vi "a前面板.vi"() -> ()   [LabVIEW 2018]
uses:
  D:/Program Files (x86)/National Instruments/LabVIEW 2018/examples/Instrument IO/Serial/support/Serial - Settings.ctl
  <vilib>/Instr/_visa.llb/VISA Configure Serial Port (Instr).vi
panel:
  out "s4":dbl format="%#.2f"
  out "s3":dbl format="%#.2f"
  out "s2":dbl format="%#.2f"
  out "s1":dbl format="%#.2f"
  out "X体横向位移2 2":dbl
  out "X体横向位移1 2":dbl
  in  "调零":bool
  out "调零后累计流量":dbl format="%.2f"
  out "瞬时流量 2":dbl format="%.2f"
  out "周向转动摩擦力2":dbl format="%#.3f"
  out "周向转动摩擦力1":dbl format="%#.3f"
  out "横向拉压力2":dbl
  out "横向拉压力1":dbl
  out "累计流量 2":dbl
  in  "VISA资源名称":refnum<visa-resource-name>="COM7"
  in  "读取前延时(ms)":u32=15
  out "响应":string
  out "读取的字节":u32
  in  "串口设置":T1={"波特率"=115200, "数据位"=8, "校验"=enum."None", "停止位"=10, "流控制"=0} {"流控制" items=["无"=0, "XON/XOFF"=1, "RTS/CTS"=2, "DTR/DSR"=4]; "停止位" items=["1.0"=10, "1.5"=15, "2.0"=20]; "数据位" min=5 max=8 step=1; "波特率" items=["75"=75, "110"=110, "134"=134, "150"=150, "300"=300, "600"=600, "1200"=1200, "1800"=1800, "2400"=2400, "4800"=4800, "7200"=7200, "9600"=9600, "14400"=14400, "19200"=19200, "28800"=28800, "38400"=38400, "56000"=56000, "57600"=57600, "115200"=115200, "128000"=128000, "230400"=230400]}
  out "连接的字符串 3":string
  out "连接的字符串 4":string
  out "瞬时流量":dbl format="%#.6f"
  out "总累计流量":dbl
  out "字符串 3":string
  out "字符串 2":string
  out "布尔 2":bool
  out "减压后气压Mpa":dbl format="%#.2f"
  in  "显示选择":bool
  out "选项卡控件":enum32{"操作面板", "数据显示面板"}(tab)
  in  "球阀预调确认":bool
  in  "球阀开口预调":dbl=0.2 min=0.0 max=100.0
  out "球阀反馈值":dbl format="%#.1f"
  in  "试验结束":bool
  in  "手动模式":bool
  in  "cns":dbl min=0.0
  in  "放气":bool
  in  "放气延迟":bool
  in  "保压时间固定":bool
  in  "不保压":bool
  in  "程序停止":bool
  out "系统通讯正常":bool
  in  "p":dbl=0.1 min=0.1
  in  "I":dbl min=0.0 max=1.0
  in  "D":dbl min=0.0 max=1.0
  in  "紧急停止":bool
  in  "电磁阀1":bool
  in  "电磁阀2":bool
  in  "球阀开口度":dbl min=0.0 max=100.0
  in  "实验所需压力Mpa":dbl=0.2 min=0.0 max=0.9
  in  "时间s":dbl=1.0 min=1.0 max=21.0
  in  "全部放气":bool
  in  "容器放气":bool
  in  "数据保存 2":bool
  in  "结束保存 2":bool
  in  "采样频率 （HZ）":dbl=1.0 min=1.0 max=1000.0
  out "采样时间计时（s）":dbl
  in  "自动模式":bool
  in  "数据保存路径":path=path "D:/data/DATA"
  out "运行状态显示":string
  in  "刷新":bool
  out "气源气压Mpa":dbl format="%.2f"
  out "容器气压 Mpa":dbl format="%#.2f"
  out "容器压力2":dbl format="%#.2f"
  out "容器压力1":dbl format="%#.2f"
  out "电磁阀2":bool
  out "球阀":dbl format="%#.2f"
  out "电磁阀1":bool
  out "管道压力2":dbl format="%#.2f"
  out "管道压力1":dbl format="%#.2f"
  in  "调零":bool
  in  "紧急停止 2":bool
  out "运行状态显示 2":string
  in  "刷新 2":bool
  in  "选项卡控件 2":enum32{"管道压力1", "管道压力2", "容器压力1", "容器压力2"}(tab)
  out "管道气压1":dbl(graph)
  out "管道压力2":dbl(graph)
  out "容器压力1":dbl(graph)
  out "容器压力2":dbl(graph)
  in  "试验结束 2":bool
  out "周向转动摩擦力1t":dbl format="%#.2f"
  out "周向转动摩擦力2t":dbl format="%#.2f"
  out "横向拉压力1t":dbl format="%#_2f"
  out "横向拉压力2t":dbl format="%#_2f"
  in  "选项卡控件 5":enum32{"力", "位移"}(tab)
  in  "选项卡控件 3":T2(tab)
  out "横向拉压力1":dbl(graph)
  out "横向拉压力2":dbl(graph)
  out "周向转动摩擦力1":dbl(graph)
  out "周向转动摩擦力2":dbl(graph)
  in  "选项卡控件 4":enum32{"X体横向位移1", "X体横向位移2", "s1-s4"}(tab)
  out "X体横向位移1":dbl(graph)
  out "X体横向位移2":dbl(graph)
  out "位移s1-s4":dynamicdata(graph)
  out "X体横向位移1t":dbl format="%#.2f"
  out "X体横向位移2t":dbl format="%#.2f"
  out "s1t":dbl format="%#.2f"
  out "s2t":dbl format="%#.2f"
  out "s3t":dbl format="%#.2f"
  out "s4t":dbl format="%#.2f"
  # "弹筒适配空间模拟试验"
  # "数据保存"
  # "自动模式"
  # "手动模式"
  # "%"
  # "%"
  # "%"
  # "Mpa"
  # "Mpa"
  # "过滤器"
  # "过滤器"
  # "手动截止阀"
  # "储气罐"
  # "目标容器"
  # "干燥机"
  # "Mpa"
  # "手动截止阀"
  # "过滤器"
  # "减压阀"
  # "Mpa"
  # "单向阀"
  # "消音器"
  # "空压机"
  # "%"
  # "手动截止阀"
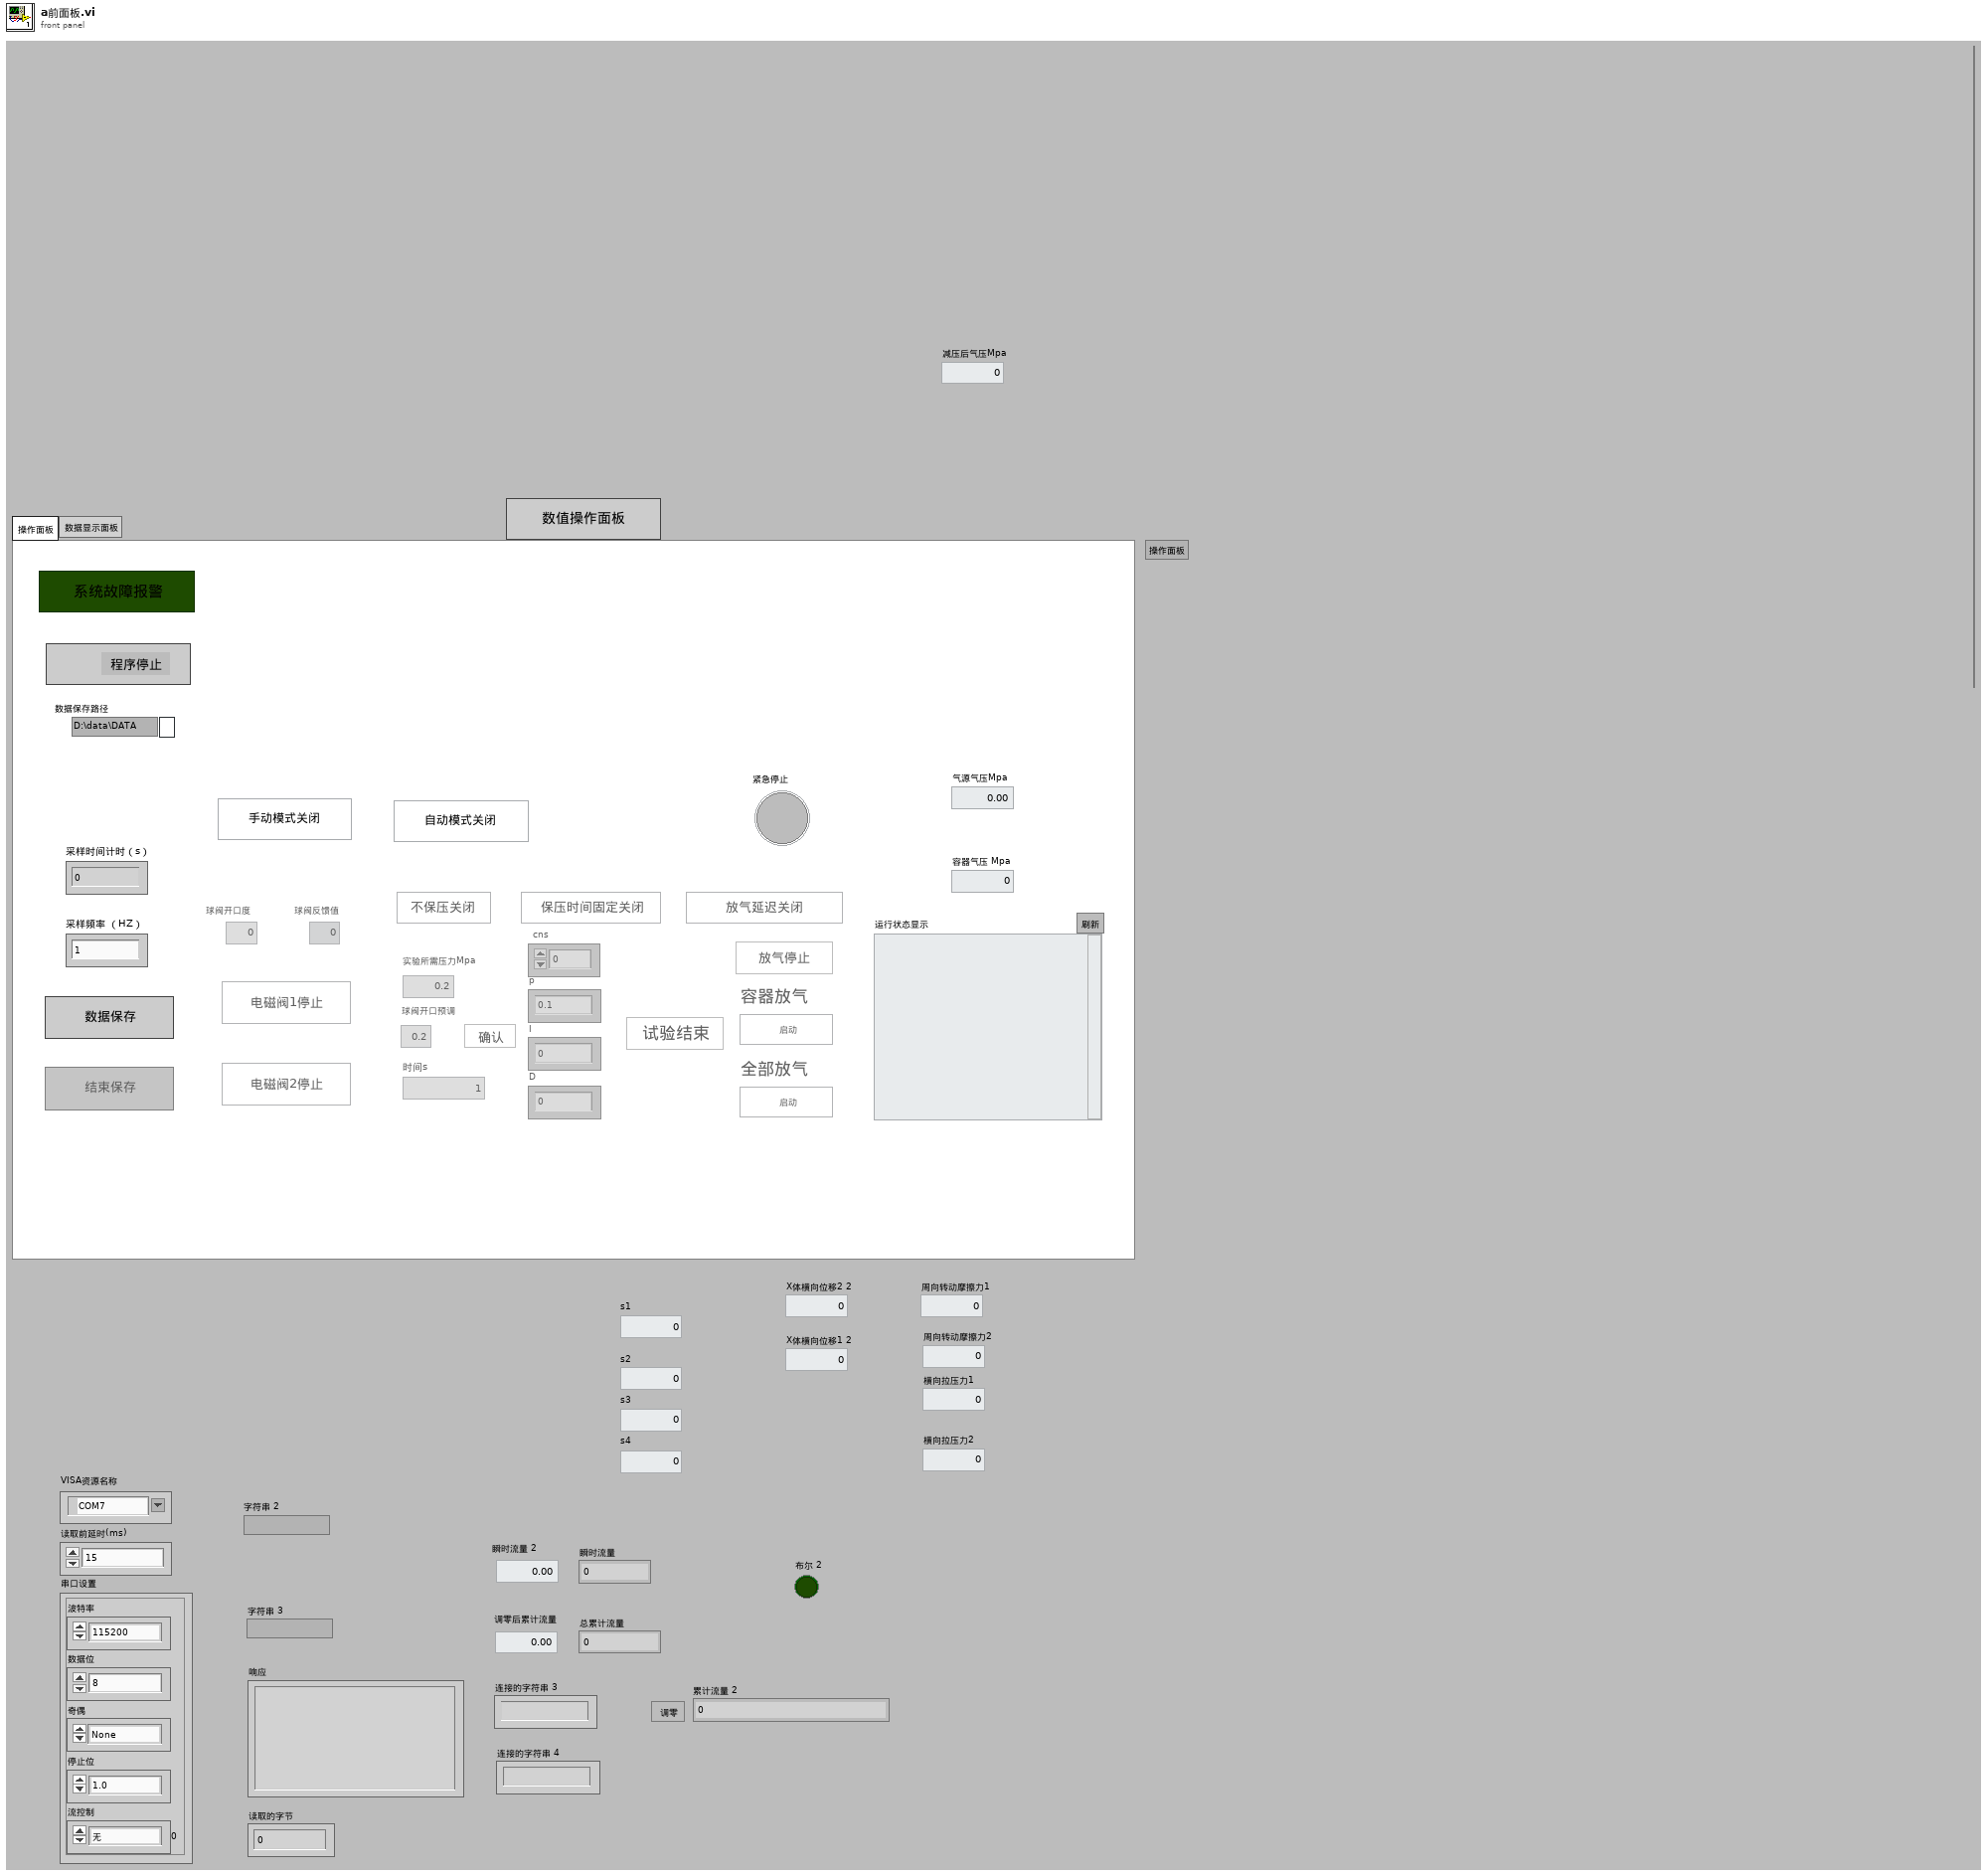
[diagram p1: front panel]
types:
  T1 = typedef "Serial - Settings.ctl" = cluster{"波特率":u32, "数据位":u16, "校验":enum16{"None", "Odd", "Even", "Mark", "Space"}, "停止位":u16, "流控制":u16}
  T2 = enum32{"横向拉压力1", "横向拉压力2", "周向转动摩擦力1", "周向转动摩擦力2"}
  T3 = enum16{"open", "replace", "create", "open or create", "replace or create", "replace or create with confirmation"}
  T4 = enum8{"Enabled", "Disabled", "Disabled and Grayed Out"}
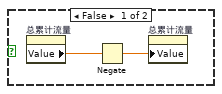
[diagram p3: hidden frame]
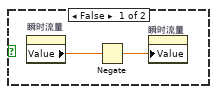
[diagram p4: hidden frame]
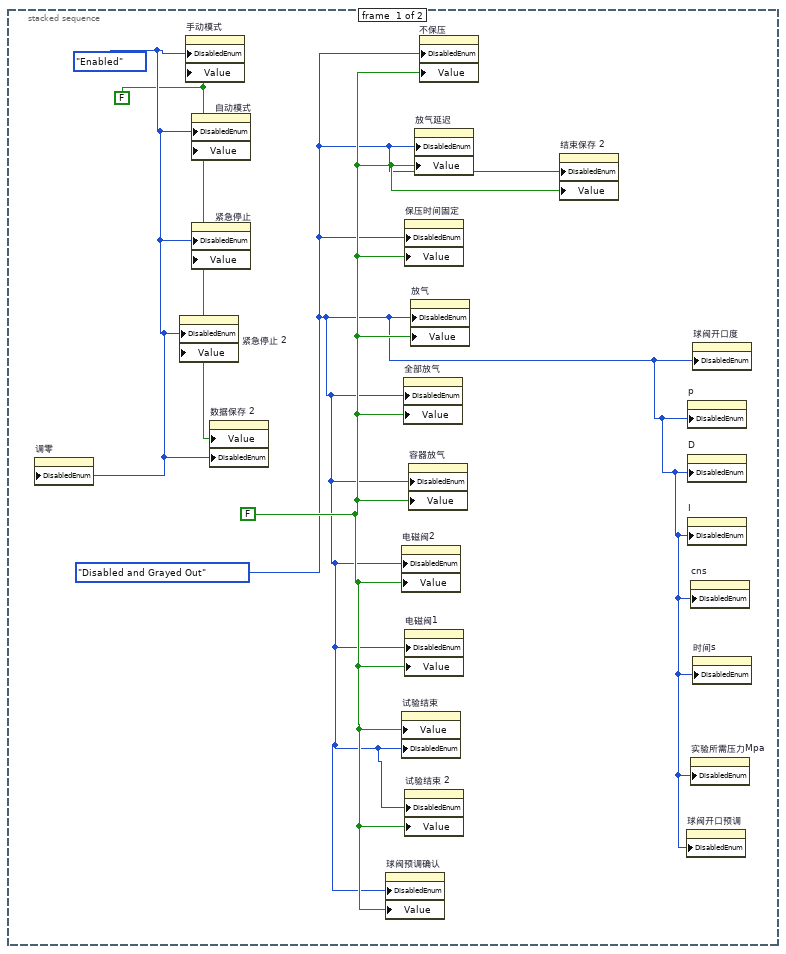
[diagram p5: hidden frame]
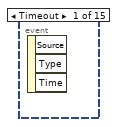
[diagram p6: hidden frame]
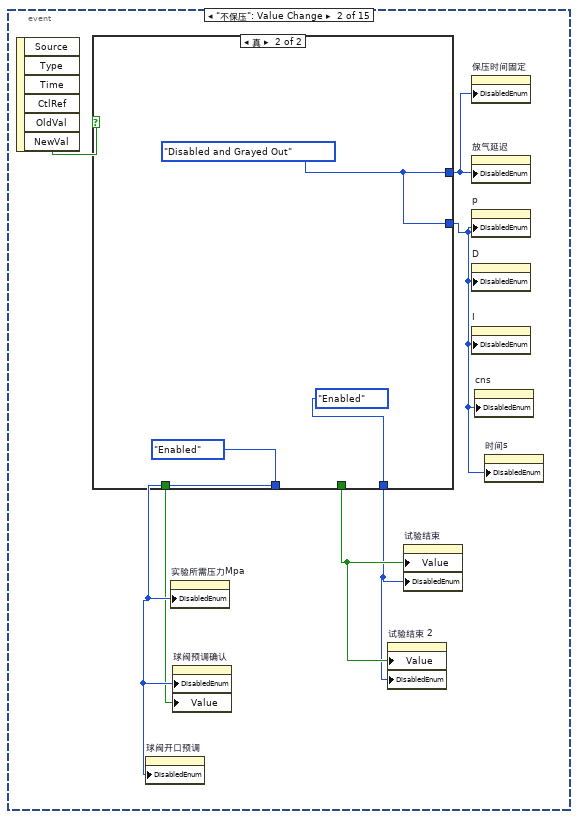
[diagram p7: hidden frame]
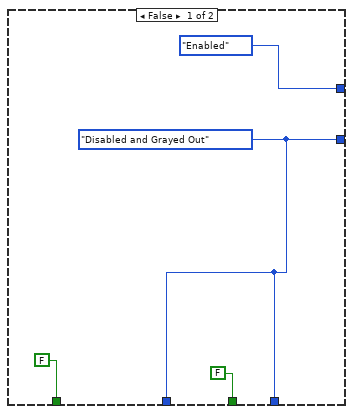
[diagram p8: hidden frame]
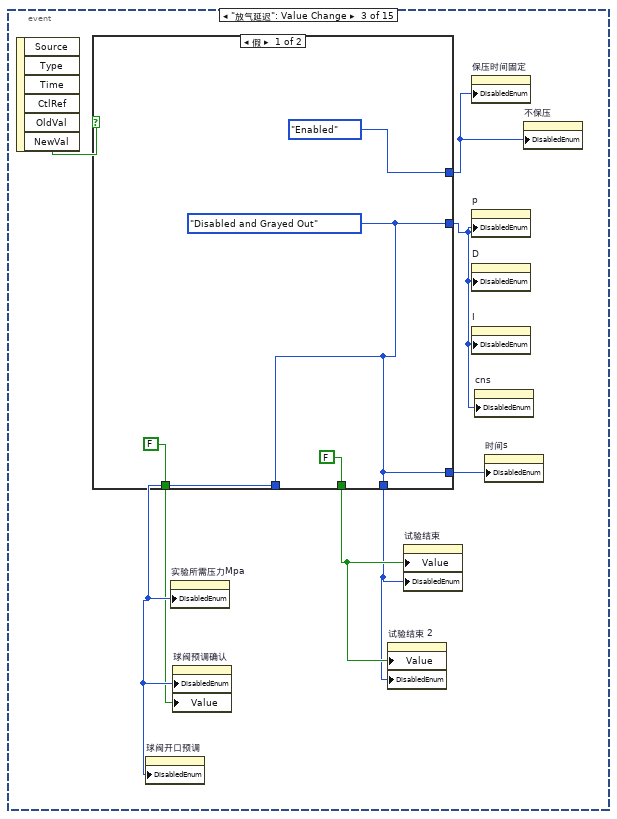
[diagram p9: hidden frame]
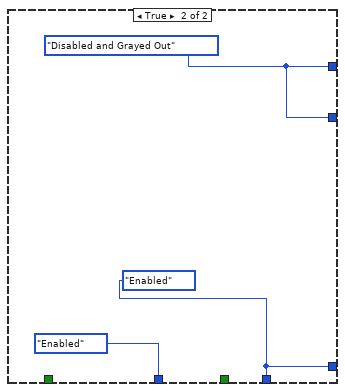
[diagram p10: hidden frame]
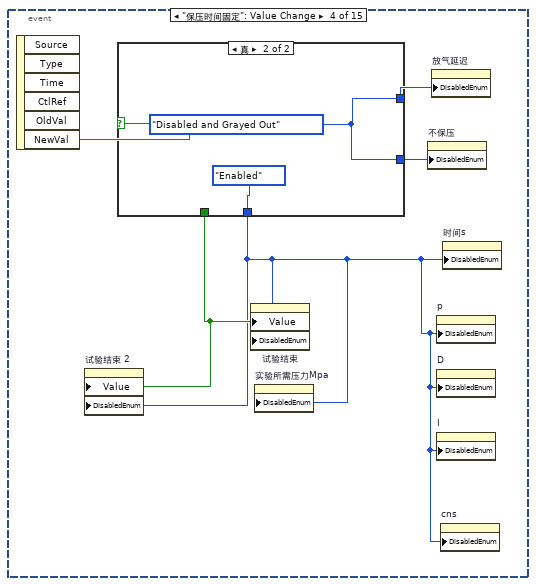
[diagram p11: hidden frame]
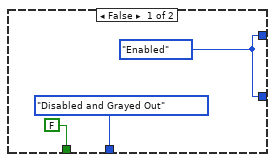
[diagram p12: hidden frame]
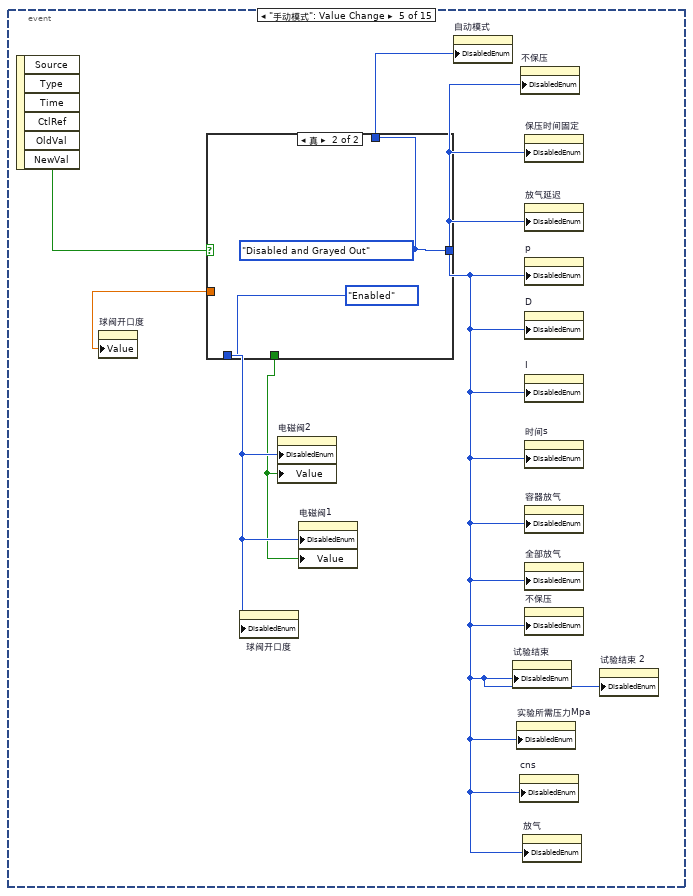
[diagram p13: hidden frame]
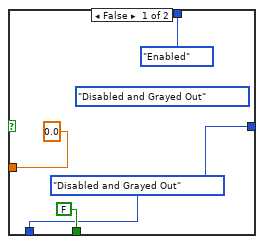
[diagram p14: hidden frame]
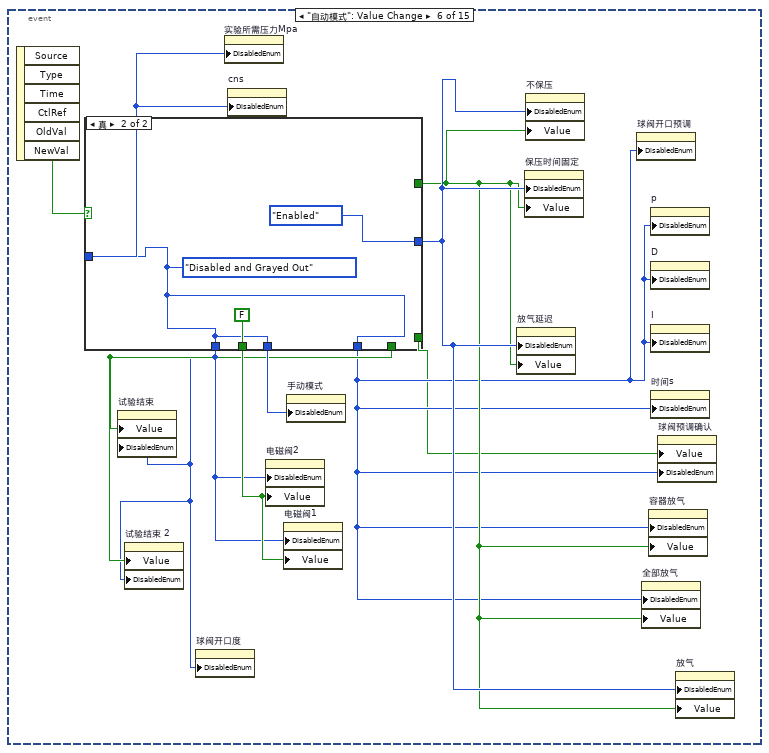
[diagram p15: hidden frame]
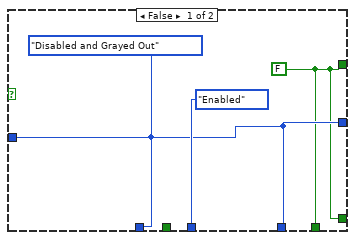
[diagram p16: hidden frame]
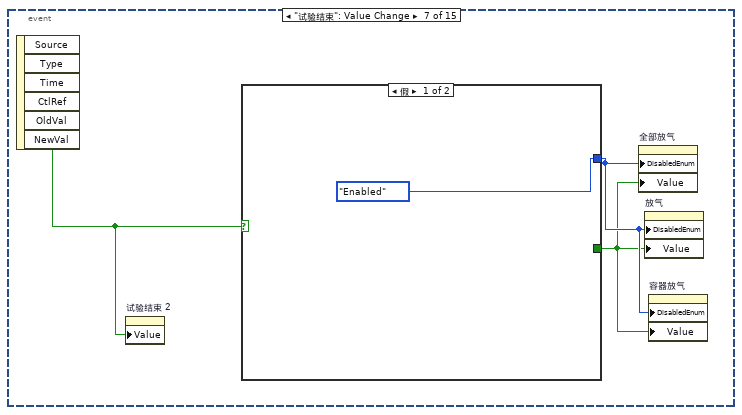
[diagram p17: hidden frame]
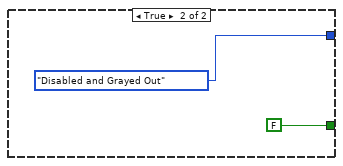
[diagram p18: hidden frame]
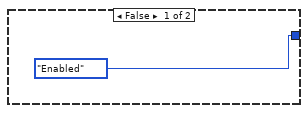
[diagram p19: hidden frame]
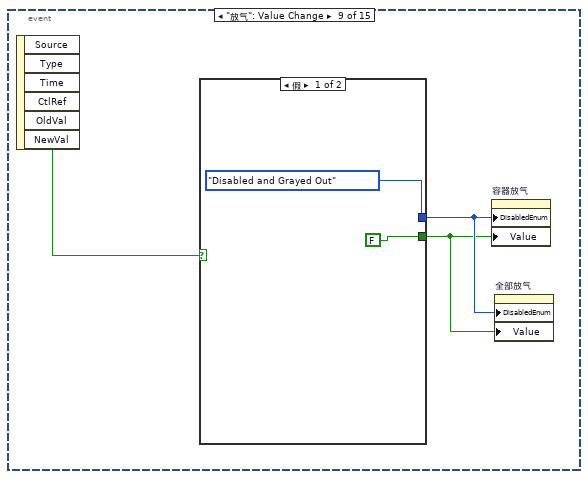
[diagram p20: hidden frame]
diagram:
  # "串口"
  # "运行状态"
  # "数据保存"
  n1 = while {
    stop <- FALSE stop-if-true
    n2 = local read "结束保存 2"() -> (w169:bool)
    n3 = Not(x=w169) -> (.not. x?=w168:bool)
    n4 = case shown="真" w168 {
      frame False {
      }
      frame True {
        n5 = case shown="真" "数据保存 2" {
          frame False {
          }
          frame True {
            n6 = flat-sequence {
              tunnel: [w195] -> w172
              tunnel: w172 -> [w196]
              frame #0 {
                w174 = "\t"
                n7 = call "数据保存表格-1.vi"("路径"="数据保存路径", "时间格式字符串(%c)"="%y年%m月%d日%H 时%M 分%S秒") -> ("添加的路径"=w195:path)
                n8 = Concatenate Strings("采样时间（s）", w174, "管道气压1(MPa)", w174, "管道气压2(MPa)", w174, "容器压力1(MPa)", w174, "容器压力2(MPa)", w174, "横向位移1", w174, "横向位移2", w174, "周向转动摩擦力1", w174, "周向转动摩擦力2", w174, "横向拉压力1", w174, "横向拉压力2", w174, "流量计瞬时流量", w174, "流量计累计流量", w174, "s1", w174, "s2", w174, "s4", w174, "s4", w174, "\r\n") -> (w193:string)
                n9 = Write to Text File(file (use dialog)=w195, text=w193) -> ()  [unwired: 2 in, 3 out]
              }
              frame #1 {
                n10 = while {
                  tunnel: w196 -> [w218]
                  i -> [w216]
                  stop <- "结束保存 2" stop-if-true
                  n11 = local read "管道压力1"() -> (w213:dbl)
                  n12 = local read "容器压力1"() -> (w211:dbl)
                  n13 = local read "周向转动摩擦力2t"() -> (w206:dbl)
                  n14 = local read "管道压力2"() -> (w212:dbl)
                  n15 = local read "容器压力2"() -> (w210:dbl)
                  n16 = local read "X体横向位移1t"() -> (w209:dbl)
                  n17 = local read "X体横向位移2t"() -> (w208:dbl)
                  n18 = local read "周向转动摩擦力1t"() -> (w207:dbl)
                  n19 = local read "横向拉压力1t"() -> (w205:dbl)
                  n20 = local read "横向拉压力2t"() -> (w204:dbl)
                  n21 = local read "瞬时流量 2"() -> (w202:dbl)
                  n22 = local read "调零后累计流量"() -> (w201:dbl)
                  n23 = local read "s4t"() -> (w197:dbl)
                  n24 = local read "s3t"() -> (w198:dbl)
                  n25 = local read "s2t"() -> (w199:dbl)
                  n26 = local read "s1t"() -> (w200:dbl)
                  n27 = Build Array(w213, w212, w211, w210, w209, w208, w207, w206, w205, w204, w202, w201, w200, w199, w198, w197) -> (w214:dbl[])
                  n28 = call "数据存储表格-2.vi"("循环次数"=w216, "数组"=w214, "频率"="采样频率 （HZ）", "file path (dialog if empty)"=w218) -> ("采样时间"=→"采样时间计时（s）":dbl)
                }
              }
            }
          }
        }
      }
    }
  }
  n29 = while {
    stop <- FALSE stop-if-true
    n30 = case shown="假" "显示选择" {
      tunnel: [enum32{"操作面板", "数据显示面板"}."操作面板" ("选项卡控件") enum32{"操作面板", "数据显示面板"}."数据显示面板" ("选项卡控件")] -> w220
      frame False {
      }
      frame True {
      }
    }
    "选项卡控件" <- w220
    n31 = Or(x="刷新", y="刷新 2") -> (x .or. y?=w221:bool)
    n32 = case shown="真" w221 {
      frame False {
      }
      frame True {
        n33 = Write to Text File(file (use dialog)=path "D:/data/state.txt" ("文件（使用对话框）"), text="   ") -> ()  [unwired: 2 in, 3 out]
      }
    }
    n34 = Read from Text File(file (use dialog)=path "D:/data/state.txt" ("文件（使用对话框）")) -> (text=→"运行状态显示" →"运行状态显示 2":string)  [unwired: 3 in, 3 out]
    n35 = flat-sequence {
      tunnel: path "D:/data" ("文件（使用对话框）") -> [w237]
      tunnel: [w236] -> w226
      tunnel: [w246] -> w228
      tunnel: [w245] -> w225
      tunnel: w226 -> [w245]
      frame #0 {
        n36 = Concatenate Strings("state" ("字符串"), ".txt" ("字符串")) -> (w243:string)
        n37 = Build Path(base path=w237, name or relative path=w243) -> (appended path=w244:path)
        n38 = Open/Create/Replace File(file path (use dialog)=w244, operation (0:open)=T3."open" ("操作(0:open)")) -> (refnum out=w239:refnum<file>)  [unwired: 4 in, 2 out]
        n39 = Set File Position(refnum=w239, from (0:start)=enum16{"start", "end", "current"}."end" ("自（0:起始）")) -> (refnum out=w236:refnum<file>)  [unwired: 2 in, 1 out]
      }
      frame #1 {
        n40 = event shown="[10] \"调零\": 值改变" {
          selector: _ -> [_ _ _ _ _ _ _ _ _ _ _ _ _ _ _ _]
          dyn-events: _ -> [_ _ _ _ _ _ _ _ _ _ _ _ _ _ _ _]
          timeout: 10 -> [_ _ _ _ _ _ _ _ _ _ _ _ _ _ _ _]
          tunnel: [_ w249 w260 w271 w281 w292 w303 w321 w340 w358 w376 w386 w404 w422 w440 w458] -> w246
          event Timeout {
            n41 = event-data() -> ()  [unwired: 1 in, 3 out]
          }
          event "数据保存 2": Value Change {
            n42 = event-data() -> ("NewVal"=w248:bool)  [unwired: 1 in, 5 out]
            n43 = case shown="假" w248 {
              tunnel: ["" w251] -> w249
              frame False {
              }
              frame True {
                n44 = Format Date/Time String(time format string (%c)="%Y/%m/%d" ("时间格式字符串(%c)")) -> (date/time string=w257:string)  [unwired: 2 in]
                n45 = Format Date/Time String(time format string (%c)="%H : %M : %S" ("时间格式字符串(%c)")) -> (date/time string=w256:string)  [unwired: 2 in]
                n46 = call <vilib>:"Space Constant.vi"() -> ("String"=w258:string)
                n47 = Concatenate Strings(w257, w258, w256, "数据保存" ("时间格式字符串(%c)"), "\r") -> (w251:string)
              }
            }
          }
          event "结束保存 2": Value Change {
            n48 = event-data() -> ("NewVal"=w259:bool)  [unwired: 1 in, 5 out]
            n49 = case shown="假" w259 {
              tunnel: ["" w262] -> w260
              frame False {
              }
              frame True {
                n50 = Format Date/Time String(time format string (%c)="%Y/%m/%d" ("时间格式字符串(%c)")) -> (date/time string=w268:string)  [unwired: 2 in]
                n51 = Format Date/Time String(time format string (%c)="%H : %M : %S" ("时间格式字符串(%c)")) -> (date/time string=w267:string)  [unwired: 2 in]
                n52 = call <vilib>:"Space Constant.vi"() -> ("String"=w269:string)
                n53 = Concatenate Strings(w268, w269, w267, "结束保存" ("时间格式字符串(%c)"), "\r") -> (w262:string)
              }
            }
          }
          event "容器放气": Value Change {
            n54 = event-data() -> ("NewVal"=w270:bool)  [unwired: 1 in, 5 out]
            n55 = case shown="假" w270 {
              tunnel: ["" w273] -> w271
              frame False {
              }
              frame True {
                n56 = Format Date/Time String(time format string (%c)="%Y/%m/%d" ("时间格式字符串(%c)")) -> (date/time string=w279:string)  [unwired: 2 in]
                n57 = Format Date/Time String(time format string (%c)="%H : %M : %S" ("时间格式字符串(%c)")) -> (date/time string=w278:string)  [unwired: 2 in]
                n58 = call <vilib>:"Space Constant.vi"() -> ("String"=w280:string)
                n59 = Concatenate Strings(w279, w280, w278, "容器放气开启" ("时间格式字符串(%c)"), "\r") -> (w273:string)
              }
            }
          }
          event "全部放气": Value Change {
            n60 = event-data() -> ("NewVal"=w282:bool)  [unwired: 1 in, 5 out]
            n61 = case shown="假" w282 {
              tunnel: ["" w284] -> w281
              frame False {
              }
              frame True {
                n62 = Format Date/Time String(time format string (%c)="%Y/%m/%d" ("时间格式字符串(%c)")) -> (date/time string=w290:string)  [unwired: 2 in]
                n63 = Format Date/Time String(time format string (%c)="%H : %M : %S" ("时间格式字符串(%c)")) -> (date/time string=w289:string)  [unwired: 2 in]
                n64 = call <vilib>:"Space Constant.vi"() -> ("String"=w291:string)
                n65 = Concatenate Strings(w290, w291, w289, "全部放气开启" ("时间格式字符串(%c)"), "\r") -> (w284:string)
              }
            }
          }
          event "放气": Value Change {
            n66 = event-data() -> ("NewVal"=w293:bool)  [unwired: 1 in, 5 out]
            n67 = case shown="假" w293 {
              tunnel: ["" w295] -> w292
              frame False {
              }
              frame True {
                n68 = Format Date/Time String(time format string (%c)="%Y/%m/%d" ("时间格式字符串(%c)")) -> (date/time string=w301:string)  [unwired: 2 in]
                n69 = Format Date/Time String(time format string (%c)="%H : %M : %S" ("时间格式字符串(%c)")) -> (date/time string=w300:string)  [unwired: 2 in]
                n70 = call <vilib>:"Space Constant.vi"() -> ("String"=w302:string)
                n71 = Concatenate Strings(w301, w302, w300, "放气模式开启" ("时间格式字符串(%c)"), "\r") -> (w295:string)
              }
            }
          }
          event "试验结束": Value Change {
            n72 = event-data() -> ("NewVal"=w304:bool)  [unwired: 1 in, 5 out]
            n73 = case shown="真" w304 {
              tunnel: [w305 w313] -> w303
              frame False {
                n74 = Format Date/Time String(time format string (%c)="%Y/%m/%d" ("时间格式字符串(%c)")) -> (date/time string=w311:string)  [unwired: 2 in]
                n75 = Format Date/Time String(time format string (%c)="%H : %M : %S" ("时间格式字符串(%c)")) -> (date/time string=w310:string)  [unwired: 2 in]
                n76 = call <vilib>:"Space Constant.vi"() -> ("String"=w312:string)
                n77 = Concatenate Strings(w311, w312, w310, "试验结束" ("时间格式字符串(%c)"), "\r") -> (w305:string)
              }
              frame True {
                n78 = Format Date/Time String(time format string (%c)="%Y/%m/%d" ("时间格式字符串(%c)")) -> (date/time string=w319:string)  [unwired: 2 in]
                n79 = Format Date/Time String(time format string (%c)="%H : %M : %S" ("时间格式字符串(%c)")) -> (date/time string=w318:string)  [unwired: 2 in]
                n80 = call <vilib>:"Space Constant.vi"() -> ("String"=w320:string)
                n81 = Concatenate Strings(w319, w320, w318, "实验开始" ("时间格式字符串(%c)"), "\r") -> (w313:string)
              }
            }
          }
          event "试验结束 2": Value Change {
            n82 = event-data() -> ("NewVal"=w322:bool)  [unwired: 1 in, 5 out]
            n83 = case shown="假" w322 {
              tunnel: [w323 w331] -> w321
              frame False {
                n84 = Format Date/Time String(time format string (%c)="%Y/%m/%d" ("时间格式字符串(%c)")) -> (date/time string=w329:string)  [unwired: 2 in]
                n85 = Format Date/Time String(time format string (%c)="%H : %M : %S" ("时间格式字符串(%c)")) -> (date/time string=w328:string)  [unwired: 2 in]
                n86 = call <vilib>:"Space Constant.vi"() -> ("String"=w330:string)
                n87 = Concatenate Strings(w329, w330, w328, "试验结束" ("时间格式字符串(%c)"), "\r") -> (w323:string)
              }
              frame True {
                n88 = Format Date/Time String(time format string (%c)="%Y/%m/%d" ("时间格式字符串(%c)")) -> (date/time string=w337:string)  [unwired: 2 in]
                n89 = Format Date/Time String(time format string (%c)="%H : %M : %S" ("时间格式字符串(%c)")) -> (date/time string=w336:string)  [unwired: 2 in]
                n90 = call <vilib>:"Space Constant.vi"() -> ("String"=w338:string)
                n91 = Concatenate Strings(w337, w338, w336, "实验开始" ("时间格式字符串(%c)"), "\r") -> (w331:string)
              }
            }
          }
          event "自动模式": Value Change {
            n92 = event-data() -> ("NewVal"=w339:bool)  [unwired: 1 in, 5 out]
            n93 = case shown="真" w339 {
              tunnel: [w342 w349] -> w340
              frame False {
                n94 = Format Date/Time String(time format string (%c)="%Y/%m/%d" ("时间格式字符串(%c)")) -> (date/time string=w341:string)  [unwired: 2 in]
                n95 = Format Date/Time String(time format string (%c)="%H : %M : %S" ("时间格式字符串(%c)")) -> (date/time string=w347:string)  [unwired: 2 in]
                n96 = call <vilib>:"Space Constant.vi"() -> ("String"=w348:string)
                n97 = Concatenate Strings(w341, w348, w347, "自动模式关闭" ("时间格式字符串(%c)"), "\r") -> (w342:string)
              }
              frame True {
                n98 = Format Date/Time String(time format string (%c)="%Y/%m/%d" ("时间格式字符串(%c)")) -> (date/time string=w355:string)  [unwired: 2 in]
                n99 = Format Date/Time String(time format string (%c)="%H : %M : %S" ("时间格式字符串(%c)")) -> (date/time string=w354:string)  [unwired: 2 in]
                n100 = call <vilib>:"Space Constant.vi"() -> ("String"=w356:string)
                n101 = Concatenate Strings(w355, w356, w354, "自动模式开启" ("时间格式字符串(%c)"), "\r") -> (w349:string)
              }
            }
          }
          event "手动模式": Value Change {
            n102 = event-data() -> ("NewVal"=w357:bool)  [unwired: 1 in, 5 out]
            n103 = case shown="假" w357 {
              tunnel: [w360 w367] -> w358
              frame False {
                n104 = Format Date/Time String(time format string (%c)="%Y/%m/%d" ("时间格式字符串(%c)")) -> (date/time string=w359:string)  [unwired: 2 in]
                n105 = Format Date/Time String(time format string (%c)="%H : %M : %S" ("时间格式字符串(%c)")) -> (date/time string=w365:string)  [unwired: 2 in]
                n106 = call <vilib>:"Space Constant.vi"() -> ("String"=w366:string)
                n107 = Concatenate Strings(w359, w366, w365, "手动模式关闭" ("时间格式字符串(%c)"), "\r") -> (w360:string)
              }
              frame True {
                n108 = Format Date/Time String(time format string (%c)="%Y/%m/%d" ("时间格式字符串(%c)")) -> (date/time string=w373:string)  [unwired: 2 in]
                n109 = Format Date/Time String(time format string (%c)="%H : %M : %S" ("时间格式字符串(%c)")) -> (date/time string=w372:string)  [unwired: 2 in]
                n110 = call <vilib>:"Space Constant.vi"() -> ("String"=w374:string)
                n111 = Concatenate Strings(w373, w374, w372, "手动模式开启" ("时间格式字符串(%c)"), "\r") -> (w367:string)
              }
            }
          }
          event "调零": Value Change {
            n112 = event-data() -> ("NewVal"=w375:bool)  [unwired: 1 in, 5 out]
            n113 = case shown="真" w375 {
              tunnel: [_ w377] -> w376
              frame False {
              }
              frame True {
                n114 = Format Date/Time String(time format string (%c)="%Y/%m/%d" ("时间格式字符串(%c)")) -> (date/time string=w383:string)  [unwired: 2 in]
                n115 = Format Date/Time String(time format string (%c)="%H : %M : %S" ("时间格式字符串(%c)")) -> (date/time string=w382:string)  [unwired: 2 in]
                n116 = call <vilib>:"Space Constant.vi"() -> ("String"=w384:string)
                n117 = Concatenate Strings(w383, w384, w382, "调零" ("时间格式字符串(%c)"), "\r") -> (w377:string)
              }
            }
          }
          event "电磁阀1": Value Change {
            n118 = event-data() -> ("NewVal"=w385:bool)  [unwired: 1 in, 5 out]
            n119 = case shown="真" w385 {
              tunnel: [w388 w395] -> w386
              frame False {
                n120 = Format Date/Time String(time format string (%c)="%Y/%m/%d" ("时间格式字符串(%c)")) -> (date/time string=w387:string)  [unwired: 2 in]
                n121 = Format Date/Time String(time format string (%c)="%H : %M : %S" ("时间格式字符串(%c)")) -> (date/time string=w393:string)  [unwired: 2 in]
                n122 = call <vilib>:"Space Constant.vi"() -> ("String"=w394:string)
                n123 = Concatenate Strings(w387, w394, w393, "电磁阀1停止" ("时间格式字符串(%c)"), "\r") -> (w388:string)
              }
              frame True {
                n124 = Format Date/Time String(time format string (%c)="%Y/%m/%d" ("时间格式字符串(%c)")) -> (date/time string=w401:string)  [unwired: 2 in]
                n125 = Format Date/Time String(time format string (%c)="%H : %M : %S" ("时间格式字符串(%c)")) -> (date/time string=w400:string)  [unwired: 2 in]
                n126 = call <vilib>:"Space Constant.vi"() -> ("String"=w402:string)
                n127 = Concatenate Strings(w401, w402, w400, "电磁阀1启动" ("时间格式字符串(%c)"), "\r") -> (w395:string)
              }
            }
          }
          event "电磁阀2": Value Change {
            n128 = event-data() -> ("NewVal"=w403:bool)  [unwired: 1 in, 5 out]
            n129 = case shown="假" w403 {
              tunnel: [w406 w413] -> w404
              frame False {
                n130 = Format Date/Time String(time format string (%c)="%Y/%m/%d" ("时间格式字符串(%c)")) -> (date/time string=w405:string)  [unwired: 2 in]
                n131 = Format Date/Time String(time format string (%c)="%H : %M : %S" ("时间格式字符串(%c)")) -> (date/time string=w411:string)  [unwired: 2 in]
                n132 = call <vilib>:"Space Constant.vi"() -> ("String"=w412:string)
                n133 = Concatenate Strings(w405, w412, w411, "电磁阀2停止" ("时间格式字符串(%c)"), "\r") -> (w406:string)
              }
              frame True {
                n134 = Format Date/Time String(time format string (%c)="%Y/%m/%d" ("时间格式字符串(%c)")) -> (date/time string=w419:string)  [unwired: 2 in]
                n135 = Format Date/Time String(time format string (%c)="%H : %M : %S" ("时间格式字符串(%c)")) -> (date/time string=w418:string)  [unwired: 2 in]
                n136 = call <vilib>:"Space Constant.vi"() -> ("String"=w420:string)
                n137 = Concatenate Strings(w419, w420, w418, "电磁阀2启动" ("时间格式字符串(%c)"), "\r") -> (w413:string)
              }
            }
          }
          event "不保压": Value Change {
            n138 = event-data() -> ("NewVal"=w421:bool)  [unwired: 1 in, 5 out]
            n139 = case shown="真" w421 {
              tunnel: [w424 w431] -> w422
              frame False {
                n140 = Format Date/Time String(time format string (%c)="%Y/%m/%d" ("时间格式字符串(%c)")) -> (date/time string=w423:string)  [unwired: 2 in]
                n141 = Format Date/Time String(time format string (%c)="%H : %M : %S" ("时间格式字符串(%c)")) -> (date/time string=w429:string)  [unwired: 2 in]
                n142 = call <vilib>:"Space Constant.vi"() -> ("String"=w430:string)
                n143 = Concatenate Strings(w423, w430, w429, "不保压模式停止" ("时间格式字符串(%c)"), "\r") -> (w424:string)
              }
              frame True {
                n144 = Format Date/Time String(time format string (%c)="%Y/%m/%d" ("时间格式字符串(%c)")) -> (date/time string=w437:string)  [unwired: 2 in]
                n145 = Format Date/Time String(time format string (%c)="%H : %M : %S" ("时间格式字符串(%c)")) -> (date/time string=w436:string)  [unwired: 2 in]
                n146 = call <vilib>:"Space Constant.vi"() -> ("String"=w438:string)
                n147 = Concatenate Strings(w437, w438, w436, "不保压模式启动" ("时间格式字符串(%c)"), "\r") -> (w431:string)
              }
            }
          }
          event "保压时间固定": Value Change {
            n148 = event-data() -> ("NewVal"=w439:bool)  [unwired: 1 in, 5 out]
            n149 = case shown="真" w439 {
              tunnel: [w442 w449] -> w440
              frame False {
                n150 = Format Date/Time String(time format string (%c)="%Y/%m/%d" ("时间格式字符串(%c)")) -> (date/time string=w441:string)  [unwired: 2 in]
                n151 = Format Date/Time String(time format string (%c)="%H : %M : %S" ("时间格式字符串(%c)")) -> (date/time string=w447:string)  [unwired: 2 in]
                n152 = call <vilib>:"Space Constant.vi"() -> ("String"=w448:string)
                n153 = Concatenate Strings(w441, w448, w447, "保压时间固定模式停止" ("时间格式字符串(%c)"), "\r") -> (w442:string)
              }
              frame True {
                n154 = Format Date/Time String(time format string (%c)="%Y/%m/%d" ("时间格式字符串(%c)")) -> (date/time string=w455:string)  [unwired: 2 in]
                n155 = Format Date/Time String(time format string (%c)="%H : %M : %S" ("时间格式字符串(%c)")) -> (date/time string=w454:string)  [unwired: 2 in]
                n156 = call <vilib>:"Space Constant.vi"() -> ("String"=w456:string)
                n157 = Concatenate Strings(w455, w456, w454, "保压时间固定模式启动" ("时间格式字符串(%c)"), "\r") -> (w449:string)
              }
            }
          }
          event "放气延迟": Value Change {
            n158 = event-data() -> ("NewVal"=w457:bool)  [unwired: 1 in, 5 out]
            n159 = case shown="假" w457 {
              tunnel: [w460 w467] -> w458
              frame False {
                n160 = Format Date/Time String(time format string (%c)="%Y/%m/%d" ("时间格式字符串(%c)")) -> (date/time string=w459:string)  [unwired: 2 in]
                n161 = Format Date/Time String(time format string (%c)="%H : %M : %S" ("时间格式字符串(%c)")) -> (date/time string=w465:string)  [unwired: 2 in]
                n162 = call <vilib>:"Space Constant.vi"() -> ("String"=w466:string)
                n163 = Concatenate Strings(w459, w466, w465, "保压时间非固定模式停止" ("时间格式字符串(%c)"), "\r") -> (w460:string)
              }
              frame True {
                n164 = Format Date/Time String(time format string (%c)="%Y/%m/%d" ("时间格式字符串(%c)")) -> (date/time string=w473:string)  [unwired: 2 in]
                n165 = Format Date/Time String(time format string (%c)="%H : %M : %S" ("时间格式字符串(%c)")) -> (date/time string=w472:string)  [unwired: 2 in]
                n166 = call <vilib>:"Space Constant.vi"() -> ("String"=w474:string)
                n167 = Concatenate Strings(w473, w474, w472, "保压时间非固定模式启动" ("时间格式字符串(%c)"), "\r") -> (w467:string)
              }
            }
          }
        }
      }
    }
    n168 = Write to Text File(file (use dialog)=w225, text=w228) -> (refnum out=w229:refnum<file>)  [unwired: 2 in, 2 out]
    n169 = Close File(refnum=w229) -> ()  [unwired: 1 in, 2 out]
  }
  n170 = Current VI's Path() -> (path=w162:path)
  n171 = Path To String(path=w162) -> (string=w164:string)
  n172 = Reverse String(1:w164) -> (0:w166:string)
  n173 = Search/Split String(string=w166, search string/char (-)="\\" ("search char (-)")) -> (match + rest of string=w165:string)  [unwired: 1 in, 2 out]
  n174 = call "xPCOpenTcpIpPort.vi"("port"="22222" ("IP Port"), "address"="192.168.0.10" ("IP Address")) -> ("error out"=w141:errorcluster, "Port"=w142:i32)
  n175 = Reverse String(1:w165) -> (0:w167:string)
  n176 = Unbundle By Name(w141) -> ("status"=w160:bool)
  n177 = Select(t="上下位机连接失败!" ("message"), s=w160, f="上下位机建立连接!" ("message")) -> (s? t:f=w157:string)
  n178 = call "xPCLoadApp.vi"("pathstr"=w167, "filename"="ce", "port"=w142) -> ("error out"=w152:errorcluster, "port copy"=w161:i32)  [unwired: 1 in]
  n179 = call "queue_message_New.vi"("message"=w157, "queue_name"="218运动系统Log Report") -> ("queue_name_copy"=w156:string)  [unwired: 1 in, 1 out]
  n180 = Unbundle By Name(w152) -> ("status"=w135:bool)
  n181 = call "xPCStartApp.vi"("port"=w161) -> ("error out"=w146:errorcluster, "port copy"=w1:i32)  [unwired: 1 in]
  n182 = Unbundle By Name(w146) -> ("status"=w149:bool)
  n183 = Select(t="控制模型下载失败!" ("message"), s=w135, f="控制模型下载成功!" ("message")) -> (s? t:f=w155:string)
  n184 = Not(x=w135) -> (.not. x?=→"系统通讯正常":bool)
  n185 = call "queue_message_New.vi"("message"=w155, "queue_name"=w156) -> ()  [unwired: 1 in, 2 out]
  n186 = Select(t="控制模型运行异常!" ("message"), s=w149, f="控制模型开始运行!" ("message")) -> (s? t:f=w148:string)
  n187 = call "queue_message_New.vi"("message"=w148) -> ()  [unwired: 2 in, 2 out]
  n188 = call "xPCGetParamIdx.vi"("blockpath"="t0" ("pathstr"), "parametername"="Value" ("filename"), "port"=w1) -> ("identifier"=w17:i32, "port copy"=w18:i32)  [unwired: 1 in, 1 out]
  n189 = call "xPCGetParamIdx.vi"("blockpath"="shoudong" ("pathstr"), "parametername"="Value" ("filename"), "port"=w1) -> ("identifier"=w48:i32, "port copy"=w47:i32)  [unwired: 1 in, 1 out]
  n190 = call "xPCGetParamIdx.vi"("blockpath"="cns" ("pathstr"), "parametername"="Value" ("filename"), "port"=w1) -> ("identifier"=w51:i32, "port copy"=w52:i32)  [unwired: 1 in, 1 out]
  n191 = call "xPCGetParamIdx.vi"("blockpath"="cns3" ("pathstr"), "parametername"="Value" ("filename"), "port"=w1) -> ("identifier"=w41:i32, "port copy"=w42:i32)  [unwired: 1 in, 1 out]
  n192 = call "xPCGetParamIdx.vi"("blockpath"="fby_qfkk" ("pathstr"), "parametername"="Value" ("filename"), "port"=w1) -> ("identifier"=w30:i32, "port copy"=w29:i32)  [unwired: 1 in, 1 out]
  n193 = call "xPCGetParamIdx.vi"("blockpath"="zidong" ("pathstr"), "parametername"="Value" ("filename"), "port"=w1) -> ("identifier"=w125:i32, "port copy"=w126:i32)  [unwired: 1 in, 1 out]
  n194 = call "xPCGetParamIdx.vi"("blockpath"="D" ("pathstr"), "parametername"="Value" ("filename"), "port"=w1) -> ("identifier"=w83:i32, "port copy"=w82:i32)  [unwired: 1 in, 1 out]
  n195 = call "xPCGetParamIdx.vi"("blockpath"="bdqy" ("pathstr"), "parametername"="Value" ("filename"), "port"=w1) -> ("identifier"=w96:i32, "port copy"=w97:i32)  [unwired: 1 in, 1 out]
  n196 = call "xPCGetParamIdx.vi"("blockpath"="P" ("pathstr"), "parametername"="Value" ("filename"), "port"=w1) -> ("identifier"=w93:i32, "port copy"=w92:i32)  [unwired: 1 in, 1 out]
  n197 = call "xPCGetParamIdx.vi"("blockpath"="time" ("pathstr"), "parametername"="Value" ("filename"), "port"=w1) -> ("identifier"=w103:i32, "port copy"=w102:i32)  [unwired: 1 in, 1 out]
  n198 = call "xPCGetParamIdx.vi"("blockpath"="I" ("pathstr"), "parametername"="Value" ("filename"), "port"=w1) -> ("identifier"=w86:i32, "port copy"=w87:i32)  [unwired: 1 in, 1 out]
  n199 = call "xPCGetParamIdx.vi"("blockpath"="jt" ("pathstr"), "parametername"="Value" ("filename"), "port"=w1) -> ("identifier"=w122:i32, "port copy"=w121:i32)  [unwired: 1 in, 1 out]
  n200 = call "xPCGetParamIdx.vi"("blockpath"="start" ("pathstr"), "parametername"="Value" ("filename"), "port"=w1) -> ("identifier"=w130:i32, "port copy"=w131:i32)  [unwired: 1 in, 1 out]
  n201 = call "xPCGetParamIdx.vi"("blockpath"="rqfq" ("pathstr"), "parametername"="Value" ("filename"), "port"=w1) -> ("identifier"=w71:i32, "port copy"=w72:i32)  [unwired: 1 in, 1 out]
  n202 = call "xPCGetParamIdx.vi"("blockpath"="qfq" ("pathstr"), "parametername"="Value" ("filename"), "port"=w1) -> ("identifier"=w78:i32, "port copy"=w77:i32)  [unwired: 1 in, 1 out]
  n203 = call "xPCGetParamIdx.vi"("blockpath"="cns2" ("pathstr"), "parametername"="Value" ("filename"), "port"=w1) -> ("identifier"=w58:i32, "port copy"=w57:i32)  [unwired: 1 in, 1 out]
  n204 = call "xPCGetParamIdx.vi"("blockpath"="cns1" ("pathstr"), "parametername"="Value" ("filename"), "port"=w1) -> ("identifier"=w61:i32, "port copy"=w62:i32)  [unwired: 1 in, 1 out]
  n205 = call "xPCGetParamIdx.vi"("blockpath"="by" ("pathstr"), "parametername"="Value" ("filename"), "port"=w1) -> ("identifier"=w112:i32, "port copy"=w111:i32)  [unwired: 1 in, 1 out]
  n206 = call "xPCGetParamIdx.vi"("blockpath"="fby" ("pathstr"), "parametername"="Value" ("filename"), "port"=w1) -> ("identifier"=w115:i32, "port copy"=w116:i32)  [unwired: 1 in, 1 out]
  n207 = call "xPCGetParamIdx.vi"("blockpath"="exp_ready" ("pathstr"), "parametername"="Value" ("filename"), "port"=w1) -> ("identifier"=w23:i32, "port copy"=w24:i32)  [unwired: 1 in, 1 out]
  n208 = call "xPCGetParamIdx.vi"("blockpath"="fq" ("pathstr"), "parametername"="Value" ("filename"), "port"=w1) -> ("identifier"=w68:i32, "port copy"=w67:i32)  [unwired: 1 in, 1 out]
  n209 = call "xPCGetParamIdx.vi"("blockpath"="fqyc" ("pathstr"), "parametername"="Value" ("filename"), "port"=w1) -> ("identifier"=w106:i32, "port copy"=w21:i32)  [unwired: 1 in, 1 out]
  n210 = while {
    tunnel: "qyyl" ("filename") -> [w777]
    tunnel: "jyf" ("filename") -> [w776]
    tunnel: "rqyl1" ("filename") -> [w775]
    tunnel: "rqyl2" ("filename") -> [w774]
    tunnel: w1 -> [w773]
    tunnel: w1 -> [w772]
    tunnel: w1 -> [w771]
    tunnel: [w767] -> w132
    tunnel: w131 -> [w765]
    tunnel: w130 -> [w764]
    shift-right: [w739] -> _
    shift-left: 0.0 -> [w762]
    tunnel: w126 -> [w745]
    tunnel: w125 -> [w744]
    shift-right: [w740] -> _
    shift-left: 0.0 -> [w743]
    tunnel: w121 -> [w735]
    tunnel: w122 -> [w736]
    shift-right: [w733] -> _
    shift-left: 0.0 -> [w738]
    tunnel: w116 -> [w730]
    tunnel: w115 -> [w729]
    shift-right: [w732] -> _
    shift-left: 0.0 -> [w727]
    tunnel: w111 -> [w723]
    tunnel: w112 -> [w724]
    shift-right: [w721] -> _
    shift-left: 0.0 -> [w726]
    tunnel: w21 -> [w718]
    tunnel: w106 -> [w717]
    shift-right: [w720] -> _
    shift-left: 0.0 -> [w715]
    tunnel: w102 -> [w711]
    tunnel: w103 -> [w712]
    shift-right: [w709] -> _
    shift-left: 0.0 -> [w714]
    tunnel: w97 -> [w706]
    tunnel: w96 -> [w705]
    shift-right: [w708] -> _
    shift-left: 0.0 -> [w703]
    tunnel: w92 -> [w699]
    tunnel: w93 -> [w700]
    shift-right: [w697] -> _
    shift-left: 0.0 -> [w702]
    tunnel: w87 -> [w694]
    tunnel: w86 -> [w693]
    shift-right: [w696] -> _
    shift-left: 0.0 -> [w658]
    tunnel: w82 -> [w688]
    tunnel: w83 -> [w689]
    shift-right: [w686] -> _
    shift-left: 0.0 -> [w691]
    tunnel: w67 -> [w663]
    tunnel: w68 -> [w664]
    shift-right: [w661] -> _
    shift-left: 0.0 -> [w666]
    tunnel: w72 -> [w670]
    tunnel: w71 -> [w669]
    shift-right: [w672] -> _
    shift-left: 0.0 -> [w667]
    tunnel: w77 -> [w675]
    tunnel: w78 -> [w676]
    shift-right: [w673] -> _
    shift-left: 0.0 -> [w678]
    tunnel: w62 -> [w654]
    tunnel: w61 -> [w653]
    shift-right: [w656] -> _
    shift-left: 0.0 -> [w651]
    tunnel: w57 -> [w647]
    tunnel: w58 -> [w648]
    shift-right: [w645] -> _
    shift-left: 0.0 -> [w650]
    tunnel: w52 -> [w642]
    tunnel: w51 -> [w640]
    shift-right: [w644] -> _
    shift-left: 0.0 -> [w639]
    tunnel: w1 -> [w638]
    tunnel: w47 -> [w629]
    tunnel: w48 -> [w630]
    shift-right: [w634] -> _
    shift-left: 0.0 -> [w631]
    tunnel: w42 -> [w627]
    tunnel: w41 -> [w625]
    shift-right: [w623] -> _
    shift-left: 0.0 -> [w624]
    tunnel: "wy1" ("filename") -> [w612]
    tunnel: "wy2" ("filename") -> [w611]
    tunnel: "5t1" ("filename") -> [w610]
    tunnel: "5t2" ("filename") -> [w609]
    tunnel: "150t1" ("filename") -> [w604]
    tunnel: "150t2" ("filename") -> [w603]
    tunnel: w1 -> [w600]
    tunnel: w1 -> [w599]
    tunnel: w1 -> [w598]
    tunnel: w1 -> [w597]
    tunnel: w1 -> [w596]
    tunnel: w1 -> [w595]
    tunnel: "qffk" ("filename") -> [w591]
    tunnel: w1 -> [w588]
    tunnel: "rqyl3" ("filename") -> [w586]
    tunnel: w1 -> [w583]
    tunnel: w29 -> [w579]
    tunnel: w30 -> [w581]
    shift-right: [w576] -> _
    shift-left: 0.0 -> [w577]
    tunnel: w24 -> [w572]
    tunnel: w23 -> [w571]
    shift-right: [w568] -> _
    shift-left: 0.0 -> [w569]
    tunnel: w18 -> [w556]
    tunnel: w17 -> [w555]
    shift-right: [w551] -> _
    shift-left: 0.0 -> [w554]
    tunnel: "t0_5t1" ("filename") -> [w550]
    tunnel: "t0_5t2" ("filename") -> [w544]
    tunnel: w1 -> [w545]
    tunnel: w1 -> [w543]
    tunnel: "t0_150t1" ("filename") -> [w542]
    tunnel: "t0_150t2" ("filename") -> [w536]
    tunnel: w1 -> [w537]
    tunnel: w1 -> [w535]
    tunnel: "t0_s1" ("filename") -> [w527]
    tunnel: w1 -> [w528]
    tunnel: "t0_wy2" ("filename") -> [w519]
    tunnel: "t0_wy1" ("filename") -> [w521]
    tunnel: w1 -> [w522]
    tunnel: w1 -> [w520]
    tunnel: "t0_s2" ("filename") -> [w511]
    tunnel: "t0_s3" ("filename") -> [w506]
    tunnel: "t0_s4" ("filename") -> [w505]
    tunnel: w1 -> [w502]
    tunnel: w1 -> [w501]
    tunnel: w1 -> [w500]
    tunnel: "s1" ("filename") -> [w499]
    tunnel: "s2" ("filename") -> [w492]
    tunnel: "s3" ("filename") -> [w491]
    tunnel: "s4" ("filename") -> [w484]
    tunnel: w1 -> [w483]
    tunnel: w1 -> [w482]
    tunnel: w1 -> [w481]
    tunnel: w1 -> [w480]
    stop <- "程序停止" stop-if-true
    n211 = call "xPCGetSigIdx.vi"("blockpath"=w591, "port"=w588) -> ("identifier"=w589:i32, "port copy"=w590:i32)  [unwired: 1 in, 1 out]
    n212 = call "xPCGetSigIdx.vi"("blockpath"=w484, "port"=w481) -> ("identifier"=w487:i32, "port copy"=w486:i32)  [unwired: 1 in, 1 out]
    n213 = call "xPCGetSigIdx.vi"("blockpath"=w505, "port"=w500) -> ("identifier"=w503:i32, "port copy"=w504:i32)  [unwired: 1 in, 1 out]
    n214 = call "xPCGetSigIdx.vi"("blockpath"=w506, "port"=w501) -> ("identifier"=w508:i32, "port copy"=w507:i32)  [unwired: 1 in, 1 out]
    n215 = call "xPCGetSigIdx.vi"("blockpath"=w775, "port"=w772) -> ("identifier"=w779:i32, "port copy"=w780:i32)  [unwired: 1 in, 1 out]
    n216 = call "xPCGetSigIdx.vi"("blockpath"=w774, "port"=w771) -> ("identifier"=w778:i32, "port copy"=w767:i32)  [unwired: 1 in, 1 out]
    n217 = call "xPCGetSigIdx.vi"("blockpath"=w491, "port"=w482) -> ("identifier"=w488:i32, "port copy"=w489:i32)  [unwired: 1 in, 1 out]
    n218 = call "xPCGetSigIdx.vi"("blockpath"=w527, "port"=w528) -> ("identifier"=w530:i32, "port copy"=w529:i32)  [unwired: 1 in, 1 out]
    n219 = call "xPCGetSigIdx.vi"("blockpath"=w499, "port"=w480) -> ("identifier"=w496:i32, "port copy"=w497:i32)  [unwired: 1 in, 1 out]
    n220 = call "xPCGetSigIdx.vi"("blockpath"=w492, "port"=w483) -> ("identifier"=w495:i32, "port copy"=w494:i32)  [unwired: 1 in, 1 out]
    n221 = call "xPCGetSigIdx.vi"("blockpath"=w550, "port"=w545) -> ("identifier"=w549:i32, "port copy"=w548:i32)  [unwired: 1 in, 1 out]
    n222 = call "xPCGetSigIdx.vi"("blockpath"=w603, "port"=w595) -> ("identifier"=w606:i32, "port copy"=w605:i32)  [unwired: 1 in, 1 out]
    n223 = call "xPCGetSigIdx.vi"("blockpath"=w511, "port"=w502) -> ("identifier"=w509:i32, "port copy"=w510:i32)  [unwired: 1 in, 1 out]
    n224 = call "xPCGetSigIdx.vi"("blockpath"=w609, "port"=w597) -> ("identifier"=w616:i32, "port copy"=w615:i32)  [unwired: 1 in, 1 out]
    n225 = call "xPCGetSigIdx.vi"("blockpath"=w544, "port"=w543) -> ("identifier"=w546:i32, "port copy"=w547:i32)  [unwired: 1 in, 1 out]
    n226 = call "xPCGetSigIdx.vi"("blockpath"=w536, "port"=w537) -> ("identifier"=w538:i32, "port copy"=w539:i32)  [unwired: 1 in, 1 out]
    n227 = call "xPCGetSigIdx.vi"("blockpath"=w611, "port"=w599) -> ("identifier"=w620:i32, "port copy"=w619:i32)  [unwired: 1 in, 1 out]
    n228 = call "xPCGetSigIdx.vi"("blockpath"=w521, "port"=w522) -> ("identifier"=w524:i32, "port copy"=w523:i32)  [unwired: 1 in, 1 out]
    n229 = call "xPCGetSigIdx.vi"("blockpath"=w610, "port"=w598) -> ("identifier"=w617:i32, "port copy"=w618:i32)  [unwired: 1 in, 1 out]
    n230 = call "xPCGetSigIdx.vi"("blockpath"=w612, "port"=w600) -> ("identifier"=w621:i32, "port copy"=w622:i32)  [unwired: 1 in, 1 out]
    n231 = call "xPCGetSigIdx.vi"("blockpath"=w519, "port"=w520) -> ("identifier"=w525:i32, "port copy"=w526:i32)  [unwired: 1 in, 1 out]
    n232 = call "xPCGetSigIdx.vi"("blockpath"=w586, "port"=w583) -> ("identifier"=w585:i32, "port copy"=w584:i32)  [unwired: 1 in, 1 out]
    n233 = call "xPCGetSigIdx.vi"("blockpath"=w777, "port"=w638) -> ("identifier"=w783:i32, "port copy"=w784:i32)  [unwired: 1 in, 1 out]
    n234 = call "xPCGetSigIdx.vi"("blockpath"=w776, "port"=w773) -> ("identifier"=w782:i32, "port copy"=w781:i32)  [unwired: 1 in, 1 out]
    n235 = call "xPCGetSigIdx.vi"("blockpath"=w604, "port"=w596) -> ("identifier"=w607:i32, "port copy"=w608:i32)  [unwired: 1 in, 1 out]
    n236 = call "xPCGetSigIdx.vi"("blockpath"=w542, "port"=w535) -> ("identifier"=w541:i32, "port copy"=w540:i32)  [unwired: 1 in, 1 out]
    n237 = Or(x="试验结束 2", y="试验结束") -> (x .or. y?=w592:bool)
    n238 = global write "全局.vi" "保压时间"("时间s") -> ()
    n239 = call "xPCGetSignal.vi"("signal"=w487, "port"=w486) -> ("Output Value"=→"s4":dbl)  [unwired: 1 in, 2 out]
    n240 = Boolean To (0,1)(Boolean=w592) -> (0, 1=w679:i16)
    n241 = Boolean To (0,1)(Boolean="放气") -> (0, 1=w660:i16)
    n242 = call "xPCGetSignal.vi"("signal"=w503, "port"=w504) -> ("Output Value"=w476:dbl)  [unwired: 1 in, 2 out]
    "s4t" <- w476
    n243 = call "xPCGetSignal.vi"("signal"=w508, "port"=w507) -> ("Output Value"=w477:dbl)  [unwired: 1 in, 2 out]
    "s3t" <- w477
    n244 = call "xPCGetSignal.vi"("signal"=w488, "port"=w489) -> ("Output Value"=→"s3":dbl)  [unwired: 1 in, 2 out]
    n245 = call "xPCGetSignal.vi"("signal"=w589, "port"=w590) -> ("Output Value"=w567:dbl)  [unwired: 1 in, 2 out]
    n246 = call "xPCGetSignal.vi"("signal"=w530, "port"=w529) -> ("Output Value"=w479:dbl)  [unwired: 1 in, 2 out]
    "s1t" <- w479
    n247 = call "xPCGetSignal.vi"("signal"=w496, "port"=w497) -> ("Output Value"=→"s1":dbl)  [unwired: 1 in, 2 out]
    n248 = call "xPCGetSignal.vi"("signal"=w495, "port"=w494) -> ("Output Value"=→"s2":dbl)  [unwired: 1 in, 2 out]
    n249 = call "xPCGetSignal.vi"("signal"=w509, "port"=w510) -> ("Output Value"=w478:dbl)  [unwired: 1 in, 2 out]
    "s2t" <- w478
    n250 = call "xPCGetSignal.vi"("signal"=w779, "port"=w780) -> ("Output Value"=→"容器压力1" →"容器压力1":dbl)  [unwired: 1 in, 2 out]
    n251 = call "xPCGetSignal.vi"("signal"=w778, "port"=w767) -> ("Output Value"=→"容器压力2" →"容器压力2":dbl)  [unwired: 1 in, 2 out]
    n252 = call "xPCGetSignal.vi"("signal"=w549, "port"=w548) -> ("Output Value"=→"周向转动摩擦力1" →"周向转动摩擦力1t":dbl)  [unwired: 1 in, 2 out]
    n253 = call "xPCGetSignal.vi"("signal"=w606, "port"=w605) -> ("Output Value"=→"横向拉压力2":dbl)  [unwired: 1 in, 2 out]
    n254 = call "xPCGetSignal.vi"("signal"=w616, "port"=w615) -> ("Output Value"=→"周向转动摩擦力2":dbl)  [unwired: 1 in, 2 out]
    n255 = call "xPCGetSignal.vi"("signal"=w546, "port"=w547) -> ("Output Value"=→"周向转动摩擦力2" →"周向转动摩擦力2t":dbl)  [unwired: 1 in, 2 out]
    n256 = call "xPCGetSignal.vi"("signal"=w538, "port"=w539) -> ("Output Value"=→"横向拉压力2" →"横向拉压力2t":dbl)  [unwired: 1 in, 2 out]
    n257 = call "xPCGetSignal.vi"("signal"=w620, "port"=w619) -> ("Output Value"=→"X体横向位移2 2":dbl)  [unwired: 1 in, 2 out]
    n258 = call "xPCGetSignal.vi"("signal"=w524, "port"=w523) -> ("Output Value"=→"X体横向位移1" →"X体横向位移1t":dbl)  [unwired: 1 in, 2 out]
    n259 = call "xPCGetSignal.vi"("signal"=w617, "port"=w618) -> ("Output Value"=→"周向转动摩擦力1":dbl)  [unwired: 1 in, 2 out]
    n260 = global write "全局.vi" "试验结束"(w679) -> ()
    n261 = call "xPCGetSignal.vi"("signal"=w621, "port"=w622) -> ("Output Value"=→"X体横向位移1 2":dbl)  [unwired: 1 in, 2 out]
    n262 = call "xPCGetSignal.vi"("signal"=w525, "port"=w526) -> ("Output Value"=→"X体横向位移2" →"X体横向位移2t":dbl)  [unwired: 1 in, 2 out]
    n263 = call "xPCGetSignal.vi"("signal"=w585, "port"=w584) -> ("Output Value"=→"容器气压 Mpa":dbl)  [unwired: 1 in, 2 out]
    n264 = call "xPCGetSignal.vi"("signal"=w783, "port"=w784) -> ("Output Value"=→"气源气压Mpa" →"管道压力1" →"管道气压1":dbl)  [unwired: 1 in, 2 out]
    n265 = call "xPCGetSignal.vi"("signal"=w782, "port"=w781) -> ("Output Value"=→"管道压力2" →"管道压力2" →"减压后气压Mpa":dbl)  [unwired: 1 in, 2 out]
    n266 = call "xPCGetSignal.vi"("signal"=w607, "port"=w608) -> ("Output Value"=→"横向拉压力1":dbl)  [unwired: 1 in, 2 out]
    n267 = call "xPCGetSignal.vi"("signal"=w541, "port"=w540) -> ("Output Value"=→"横向拉压力1" →"横向拉压力1t":dbl)  [unwired: 1 in, 2 out]
    n268 = global write "全局.vi" "放气"(w660) -> ()
    n269 = Or(x="紧急停止", y="紧急停止 2") -> (x .or. y?=w747:bool)
    n270 = Boolean To (0,1)(Boolean=w747) -> (0, 1=w748:i16)
    n271 = global read "全局.vi" "拉压力调零"() -> (w551:dbl)
    n272 = global read "全局.vi" "球阀开口度 预调"() -> (w576:dbl)
    n273 = global read "全局.vi" "球阀 开口度"() -> (w623:dbl)
    n274 = global read "全局.vi" "实验所需气压"() -> (w708:dbl)
    n275 = global write "全局.vi" "球阀反馈值"(w567) -> ()
    n276 = global write "全局.vi" "紧急停止"(w748) -> ()
    n277 = global read "全局.vi" "保压时间"() -> (w709:dbl)
    n278 = global read "全局.vi" "cns"() -> (w644:dbl)
    n279 = global read "全局.vi" "D"() -> (w686:dbl)
    n280 = global read "全局.vi" "P"() -> (w697:dbl)
    n281 = global read "全局.vi" "I"() -> (w696:dbl)
    n282 = global read "全局.vi" "保压时间固定"() -> (w721:dbl)
    n283 = Boolean To (0,1)(Boolean="全部放气") -> (0, 1=w755:i16)
    n284 = Boolean To (0,1)(Boolean="电磁阀1") -> (0, 1=w752:i16)
    n285 = global read "全局.vi" "手动模式"() -> (w634:dbl)
    n286 = global read "全局.vi" "球阀预调确认"() -> (w568:dbl)
    n287 = global read "全局.vi" "容器放气"() -> (w672:dbl)
    n288 = global read "全局.vi" "全部放气"() -> (w673:dbl)
    n289 = global read "全局.vi" "电磁阀2"() -> (w645:dbl)
    n290 = global read "全局.vi" "放气延迟"() -> (w720:dbl)
    n291 = global read "全局.vi" "电磁阀1"() -> (w656:dbl)
    n292 = global read "全局.vi" "紧急停止"() -> (w733:dbl)
    n293 = global read "全局.vi" "自动模式"() -> (w740:dbl)
    n294 = global read "全局.vi" "试验结束"() -> (w739:dbl)
    n295 = global write "全局.vi" "实验所需气压"("实验所需压力Mpa") -> ()
    n296 = global read "全局.vi" "不保压"() -> (w732:dbl)
    n297 = Multiply(x=20.0, y=w567) -> (x*y=→"球阀反馈值" →"球阀":dbl)
    n298 = global read "全局.vi" "放气"() -> (w661:dbl)
    n299 = global write "全局.vi" "全部放气"(w755) -> ()
    n300 = global write "全局.vi" "电磁阀1"(w752) -> ()
    n301 = Not Equal?(x=w639, y=w644) -> (x != y?=w641:bool)
    n302 = Build Array(w576) -> (w578:dbl[])
    n303 = Build Array(w644) -> (w643:dbl[])
    n304 = Not Equal?(x=w624, y=w623) -> (x != y?=w626:bool)
    n305 = Not Equal?(x=w577, y=w576) -> (x != y?=w580:bool)
    n306 = Build Array(w623) -> (w628:dbl[])
    n307 = Not Equal?(x=w691, y=w686) -> (x != y?=w690:bool)
    n308 = Build Array(w686) -> (w687:dbl[])
    n309 = Not Equal?(x=w703, y=w708) -> (x != y?=w704:bool)
    n310 = Build Array(w708) -> (w707:dbl[])
    n311 = Not Equal?(x=w702, y=w697) -> (x != y?=w701:bool)
    n312 = Not Equal?(x=w714, y=w709) -> (x != y?=w713:bool)
    n313 = Build Array(w697) -> (w698:dbl[])
    n314 = Not Equal?(x=w658, y=w696) -> (x != y?=w692:bool)
    n315 = Build Array(w709) -> (w710:dbl[])
    n316 = Build Array(w696) -> (w695:dbl[])
    n317 = Boolean To (0,1)(Boolean="调零") -> (0, 1=w558:i16)
    n318 = Not Equal?(x=w554, y=w551) -> (x != y?=w553:bool)
    n319 = Build Array(w551) -> (w552:dbl[])
    n320 = Not Equal?(x=w631, y=w634) -> (x != y?=w632:bool)
    n321 = Build Array(w634) -> (w633:dbl[])
    n322 = Not Equal?(x=w667, y=w672) -> (x != y?=w668:bool)
    n323 = Build Array(w672) -> (w671:dbl[])
    n324 = Not Equal?(x=w678, y=w673) -> (x != y?=w677:bool)
    n325 = Not Equal?(x=w726, y=w721) -> (x != y?=w725:bool)
    n326 = Build Array(w673) -> (w674:dbl[])
    n327 = Not Equal?(x=w650, y=w645) -> (x != y?=w649:bool)
    n328 = Build Array(w721) -> (w722:dbl[])
    n329 = Build Array(w645) -> (w646:dbl[])
    n330 = Not Equal?(x=w666, y=w661) -> (x != y?=w665:bool)
    n331 = Not Equal?(x=w651, y=w656) -> (x != y?=w652:bool)
    n332 = Not Equal?(x=w743, y=w740) -> (x != y?=w742:bool)
    n333 = Not Equal?(x=w715, y=w720) -> (x != y?=w716:bool)
    n334 = Build Array(w661) -> (w662:dbl[])
    n335 = Build Array(w656) -> (w655:dbl[])
    n336 = Build Array(w740) -> (w741:dbl[])
    n337 = Build Array(w720) -> (w719:dbl[])
    n338 = Not Equal?(x=w762, y=w739) -> (x != y?=w763:bool)
    n339 = Merge Signals(w479, w478, w477, w476) -> (→"位移s1-s4":dynamicdata)
    n340 = Build Array(w739) -> (w766:dbl[])
    n341 = Not Equal?(x=w738, y=w733) -> (x != y?=w737:bool)
    n342 = Not Equal?(x=w727, y=w732) -> (x != y?=w728:bool)
    n343 = Build Array(w733) -> (w734:dbl[])
    n344 = Build Array(w732) -> (w731:dbl[])
    n345 = Not Equal?(x=w569, y=w568) -> (x != y?=w570:bool)
    n346 = Build Array(w568) -> (w573:dbl[])
    n347 = global write "全局.vi" "拉压力调零"(w558) -> ()
    n348 = Boolean To (0,1)(Boolean="容器放气") -> (0, 1=w754:i16)
    n349 = case shown="真" w641 {
      tunnel: w643 -> [_ w801]
      tunnel: w642 -> [_ w802]
      tunnel: w640 -> [_ w800]
      frame False {
      }
      frame True {
        n350 = call "xPCSetParam.vi"("value"=w801, "index"=w800, "port"=w802) -> ()  [unwired: 1 in, 2 out]
      }
    }
    n351 = case shown="真" w626 {
      tunnel: w628 -> [_ w794]
      tunnel: w627 -> [_ w796]
      tunnel: w625 -> [_ w795]
      frame False {
      }
      frame True {
        n352 = call "xPCSetParam.vi"("value"=w794, "index"=w795, "port"=w796) -> ()  [unwired: 1 in, 2 out]
      }
    }
    n353 = case shown="真" w580 {
      tunnel: w578 -> [_ w791]
      tunnel: w579 -> [_ w793]
      tunnel: w581 -> [_ w792]
      frame False {
      }
      frame True {
        n354 = call "xPCSetParam.vi"("value"=w791, "index"=w792, "port"=w793) -> ()  [unwired: 1 in, 2 out]
      }
    }
    n355 = Boolean To (0,1)(Boolean="电磁阀2") -> (0, 1=w751:i16)
    n356 = case shown="真" w690 {
      tunnel: w687 -> [_ w818]
      tunnel: w688 -> [_ w820]
      tunnel: w689 -> [_ w819]
      frame False {
      }
      frame True {
        n357 = call "xPCSetParam.vi"("value"=w818, "index"=w819, "port"=w820) -> ()  [unwired: 1 in, 2 out]
      }
    }
    n358 = case shown="真" w704 {
      tunnel: w707 -> [_ w827]
      tunnel: w706 -> [_ w829]
      tunnel: w705 -> [_ w828]
      frame False {
      }
      frame True {
        n359 = call "xPCSetParam.vi"("value"=w827, "index"=w828, "port"=w829) -> ()  [unwired: 1 in, 2 out]
      }
    }
    n360 = case shown="真" w701 {
      tunnel: w698 -> [_ w824]
      tunnel: w699 -> [_ w826]
      tunnel: w700 -> [_ w825]
      frame False {
      }
      frame True {
        n361 = call "xPCSetParam.vi"("value"=w824, "index"=w825, "port"=w826) -> ()  [unwired: 1 in, 2 out]
      }
    }
    n362 = case shown="真" w713 {
      tunnel: w710 -> [_ w830]
      tunnel: w711 -> [_ w832]
      tunnel: w712 -> [_ w831]
      frame False {
      }
      frame True {
        n363 = call "xPCSetParam.vi"("value"=w830, "index"=w831, "port"=w832) -> ()  [unwired: 1 in, 2 out]
      }
    }
    n364 = case shown="真" w692 {
      tunnel: w695 -> [_ w821]
      tunnel: w694 -> [_ w823]
      tunnel: w693 -> [_ w822]
      frame False {
      }
      frame True {
        n365 = call "xPCSetParam.vi"("value"=w821, "index"=w822, "port"=w823) -> ()  [unwired: 1 in, 2 out]
      }
    }
    n366 = global write "全局.vi" "P"("p") -> ()
    n367 = case shown="真" w553 {
      tunnel: w556 -> [_ w787]
      tunnel: w555 -> [_ w786]
      tunnel: w552 -> [_ w785]
      frame False {
      }
      frame True {
        n368 = call "xPCSetParam.vi"("value"=w785, "index"=w786, "port"=w787) -> ()  [unwired: 1 in, 2 out]
      }
    }
    n369 = case shown="真" w632 {
      tunnel: w629 -> [_ w799]
      tunnel: w630 -> [_ w798]
      tunnel: w633 -> [_ w797]
      frame False {
      }
      frame True {
        n370 = call "xPCSetParam.vi"("value"=w797, "index"=w798, "port"=w799) -> ()  [unwired: 1 in, 2 out]
      }
    }
    n371 = global write "全局.vi" "电磁阀2"(w751) -> ()
    n372 = global write "全局.vi" "容器放气"(w754) -> ()
    n373 = case shown="真" w668 {
      tunnel: w671 -> [_ w812]
      tunnel: w670 -> [_ w814]
      tunnel: w669 -> [_ w813]
      frame False {
      }
      frame True {
        n374 = call "xPCSetParam.vi"("value"=w812, "index"=w813, "port"=w814) -> ()  [unwired: 1 in, 2 out]
      }
    }
    n375 = case shown="真" w742 {
      tunnel: w745 -> [_ w847]
      tunnel: w744 -> [_ w846]
      tunnel: w741 -> [_ w845]
      frame False {
      }
      frame True {
        n376 = call "xPCSetParam.vi"("value"=w845, "index"=w846, "port"=w847) -> ()  [unwired: 1 in, 2 out]
      }
    }
    n377 = case shown="真" w677 {
      tunnel: w674 -> [_ w809]
      tunnel: w675 -> [_ w811]
      tunnel: w676 -> [_ w810]
      frame False {
      }
      frame True {
        n378 = call "xPCSetParam.vi"("value"=w809, "index"=w810, "port"=w811) -> ()  [unwired: 1 in, 2 out]
      }
    }
    n379 = case shown="真" w725 {
      tunnel: w722 -> [_ w836]
      tunnel: w723 -> [_ w838]
      tunnel: w724 -> [_ w837]
      frame False {
      }
      frame True {
        n380 = call "xPCSetParam.vi"("value"=w836, "index"=w837, "port"=w838) -> ()  [unwired: 1 in, 2 out]
      }
    }
    n381 = case shown="真" w649 {
      tunnel: w646 -> [_ w803]
      tunnel: w647 -> [_ w805]
      tunnel: w648 -> [_ w804]
      frame False {
      }
      frame True {
        n382 = call "xPCSetParam.vi"("value"=w803, "index"=w804, "port"=w805) -> ()  [unwired: 1 in, 2 out]
      }
    }
    n383 = case shown="真" w665 {
      tunnel: w662 -> [_ w815]
      tunnel: w663 -> [_ w817]
      tunnel: w664 -> [_ w816]
      frame False {
      }
      frame True {
        n384 = call "xPCSetParam.vi"("value"=w815, "index"=w816, "port"=w817) -> ()  [unwired: 1 in, 2 out]
      }
    }
    n385 = case shown="真" w652 {
      tunnel: w655 -> [_ w806]
      tunnel: w654 -> [_ w808]
      tunnel: w653 -> [_ w807]
      frame False {
      }
      frame True {
        n386 = call "xPCSetParam.vi"("value"=w806, "index"=w807, "port"=w808) -> ()  [unwired: 1 in, 2 out]
      }
    }
    n387 = case shown="真" w716 {
      tunnel: w719 -> [_ w833]
      tunnel: w718 -> [_ w835]
      tunnel: w717 -> [_ w834]
      frame False {
      }
      frame True {
        n388 = call "xPCSetParam.vi"("value"=w833, "index"=w834, "port"=w835) -> ()  [unwired: 1 in, 2 out]
      }
    }
    n389 = case shown="真" w763 {
      tunnel: w766 -> [_ w848]
      tunnel: w765 -> [_ w850]
      tunnel: w764 -> [_ w849]
      frame False {
      }
      frame True {
        n390 = call "xPCSetParam.vi"("value"=w848, "index"=w849, "port"=w850) -> ()  [unwired: 1 in, 2 out]
      }
    }
    n391 = case shown="真" w737 {
      tunnel: w734 -> [_ w842]
      tunnel: w735 -> [_ w844]
      tunnel: w736 -> [_ w843]
      frame False {
      }
      frame True {
        n392 = call "xPCSetParam.vi"("value"=w842, "index"=w843, "port"=w844) -> ()  [unwired: 1 in, 2 out]
      }
    }
    n393 = case shown="真" w728 {
      tunnel: w731 -> [_ w839]
      tunnel: w730 -> [_ w841]
      tunnel: w729 -> [_ w840]
      frame False {
      }
      frame True {
        n394 = call "xPCSetParam.vi"("value"=w839, "index"=w840, "port"=w841) -> ()  [unwired: 1 in, 2 out]
      }
    }
    n395 = case shown="真" w570 {
      tunnel: w573 -> [_ w788]
      tunnel: w572 -> [_ w790]
      tunnel: w571 -> [_ w789]
      frame False {
      }
      frame True {
        n396 = call "xPCSetParam.vi"("value"=w788, "index"=w789, "port"=w790) -> ()  [unwired: 1 in, 2 out]
      }
    }
    n397 = global write "全局.vi" "I"("I") -> ()
    n398 = Boolean To (0,1)(Boolean="手动模式") -> (0, 1=w636:i16)
    n399 = Boolean To (0,1)(Boolean="自动模式") -> (0, 1=w753:i16)
    n400 = Boolean To (0,1)(Boolean="不保压") -> (0, 1=w684:i16)
    n401 = global write "全局.vi" "手动模式"(w636) -> ()
    n402 = global write "全局.vi" "自动模式"(w753) -> ()
    n403 = global write "全局.vi" "不保压"(w684) -> ()
    n404 = global write "全局.vi" "D"("D") -> ()
    n405 = Multiply(x=0.05, y="球阀开口预调") -> (x*y=w560:dbl)
    n406 = global write "全局.vi" "球阀开口度 预调"(w560) -> ()
    n407 = Multiply(x=0.05, y="球阀开口度") -> (x*y=w563:dbl)
    n408 = Boolean To (0,1)(Boolean="放气延迟") -> (0, 1=w682:i16)
    n409 = Boolean To (0,1)(Boolean="保压时间固定") -> (0, 1=w680:i16)
    n410 = Boolean To (0,1)(Boolean="球阀预调确认") -> (0, 1=w575:i16)
    n411 = global write "全局.vi" "球阀 开口度"(w563) -> ()
    n412 = global write "全局.vi" "保压时间固定"(w680) -> ()
    n413 = global write "全局.vi" "放气延迟"(w682) -> ()
    n414 = global write "全局.vi" "球阀预调确认"(w575) -> ()
    n415 = global write "全局.vi" "布尔"("程序停止") -> ()
    n416 = global write "全局.vi" "cns"("cns") -> ()
    "布尔 2" <- "程序停止"
    "电磁阀1" <- "电磁阀1"
    "电磁阀2" <- "电磁阀2"
  }
  n417 = stacked-sequence {
    tunnel: w132 -> [w851 _]
    frame #0 {
      n418 = call "xPCStopApp.vi"("port"=w851) -> ("port copy"=w852:i32)  [unwired: 1 in, 1 out]
      n419 = call "xPCClosePort.vi"("port"=w852) -> ()  [unwired: 1 in, 2 out]
    }
    frame #1 {
      n420 = global read "全局.vi" "布尔"() -> (w853:bool)
      n421 = Stop(stop? (T)=w853) -> ()
    }
  }
  n422 = while {
    stop <- FALSE stop-if-true
    n423 = local read "连接的字符串 3"() -> (w867:string)
    n424 = String To Byte Array(string=w867) -> (unsigned byte array=w869:u8[])
    n425 = for {
      shift-right: [w992] -> w868
      shift-left: "" -> [w994]
      tunnel: w869 -> [w1001] mode=indexing
      n426 = Number To Hexadecimal String(2:w1001) -> (0:w995:string)  [unwired: 1 in]
      n427 = String Length(string=w995) -> (length=w1000:i32)
      n428 = Concatenate Strings("" ("字符串"), w995) -> (w996:string)
      n429 = Equal?(x=w1000, y=2) -> (x = y?=w998:bool)
      n430 = Select(t=w995, s=w998, f=w996) -> (s? t:f=w993:string)
      n431 = Concatenate Strings(w994, w993) -> (w992:string)
    }
    "字符串 2" <- w868
    n432 = flat-sequence {
      tunnel: [w951] -> w862
      tunnel: w862 -> [w957]
      tunnel: [w957] -> w861
      tunnel: w861 -> [w969]
      tunnel: [w969] -> w860
      tunnel: [w961] -> w859
      tunnel: w860 -> [w981]
      tunnel: w859 -> [w975]
      frame #0 {
        # "删除要转换的字符串所有空格，然后转换成二进制"
        n433 = local read "字符串 2"() -> (w947:string)
        n434 = call <vilib>:"Space Constant.vi"() -> ("String"=w950:string)
        n435 = Search and Replace String(replace all?=TRUE ("替换全部？(F)"), input string=w947, search string=w950) -> (result string=w948:string)  [unwired: 5 in, 3 out]
        n436 = call "16转2进制字符串.vi"("16进制字符串"=w948) -> ("转换后二进制字符"=w951:string)
      }
      frame #1 {
        # "提取第一位用于判断正负"
        n437 = String Subset(string=w957, offset (0)=0 ("偏移量(0)"), length (rest)=1 ("长度（剩余）")) -> (substring=w953:string)
        n438 = Equal?(x=w953, y="0") -> (x = y?=w955:bool)
        n439 = case shown="真" w955 {
          frame False {
            n440 = property on="瞬时流量" class="DigNum (严格)"() -> ("Value"=w959:dbl)  [unwired: 2 in, 2 out]
            n441 = Negate(x=w959) -> (-x=w958:dbl)
            n442 = property on="瞬时流量" class="DigNum (严格)"("Value"=w958) -> ()  [unwired: 2 in, 2 out]
          }
          frame True {
            n443 = property on="瞬时流量" class="DigNum (严格)"() -> ("Value"=w960:dbl)  [unwired: 2 in, 2 out]
            n444 = property on="瞬时流量" class="DigNum (严格)"("Value"=w960) -> ()  [unwired: 2 in, 2 out]
          }
        }
      }
      frame #2 {
        # "提取第2到9位阶码，用于计算2^（E-127）"
        n445 = String Subset(string=w969, offset (0)=1 ("偏移量(0)"), length (rest)=8 ("长度（剩余）")) -> (substring=w966:string)
        n446 = call "2转10进制字符串.vi"("二进制字符串"=w966) -> ("十进制数值"=w967:i32)
        n447 = Subtract(x=w967, y=127) -> (x-y=w968:i32)
        n448 = Scale By Power Of 2(n=w968, x=sgl 1.0 ("长度（剩余）")) -> (x*2^n=w961:sgl)
      }
      frame #3 {
        # "提取最后23位，用于计算1+M/2^23"
        n449 = String Subset(string=w981, offset (0)=9 ("偏移量(0)")) -> (substring=w976:string)  [unwired: 1 in]
        n450 = call "2转10进制字符串.vi"("二进制字符串"=w976) -> ("十进制数值"=w980:i32)
        n451 = Scale By Power Of 2(n=i16 23, x=sgl 1.0 ("长度（剩余）")) -> (x*2^n=w977:sgl)
        n452 = Divide(x=w980, y=w977) -> (x/y=w978:sgl)
        n453 = Add(x=w978, y=1.0) -> (x+y=w979:dbl)
        n454 = Multiply(x=w979, y=w975) -> (x*y=→"瞬时流量" →"瞬时流量 2":dbl)
      }
    }
    n455 = flat-sequence {
      tunnel: [w916] -> w858
      tunnel: w858 -> [w922]
      tunnel: [w922] -> w857
      tunnel: w857 -> [w934]
      tunnel: [w934] -> w856
      tunnel: [w926] -> w855
      tunnel: w856 -> [w946]
      tunnel: w855 -> [w939]
      frame #0 {
        # "删除要转换的字符串所有空格，然后转换成二进制"
        n456 = local read "字符串 3"() -> (w912:string)
        n457 = call <vilib>:"Space Constant.vi"() -> ("String"=w915:string)
        n458 = Search and Replace String(replace all?=TRUE ("替换全部？(F)"), input string=w912, search string=w915) -> (result string=w913:string)  [unwired: 5 in, 3 out]
        n459 = call "16转2进制字符串.vi"("16进制字符串"=w913) -> ("转换后二进制字符"=w916:string)
      }
      frame #1 {
        # "提取第一位用于判断正负"
        n460 = String Subset(string=w922, offset (0)=0 ("偏移量(0)"), length (rest)=1 ("长度（剩余）")) -> (substring=w918:string)
        n461 = Equal?(x=w918, y="0") -> (x = y?=w920:bool)
        n462 = case shown="真" w920 {
          frame False {
            n463 = property on="总累计流量" class="DigNum (严格)"() -> ("Value"=w924:dbl)  [unwired: 2 in, 2 out]
            n464 = Negate(x=w924) -> (-x=w923:dbl)
            n465 = property on="总累计流量" class="DigNum (严格)"("Value"=w923) -> ()  [unwired: 2 in, 2 out]
          }
          frame True {
            n466 = property on="总累计流量" class="DigNum (严格)"() -> ("Value"=w925:dbl)  [unwired: 2 in, 2 out]
            n467 = property on="总累计流量" class="DigNum (严格)"("Value"=w925) -> ()  [unwired: 2 in, 2 out]
          }
        }
      }
      frame #2 {
        # "提取第2到9位阶码，用于计算2^（E-127）"
        n468 = String Subset(string=w934, offset (0)=1 ("偏移量(0)"), length (rest)=8 ("长度（剩余）")) -> (substring=w931:string)
        n469 = call "2转10进制字符串.vi"("二进制字符串"=w931) -> ("十进制数值"=w932:i32)
        n470 = Subtract(x=w932, y=127) -> (x-y=w933:i32)
        n471 = Scale By Power Of 2(n=w933, x=sgl 1.0 ("长度（剩余）")) -> (x*2^n=w926:sgl)
      }
      frame #3 {
        # "提取最后23位，用于计算1+M/2^23"
        n472 = String Subset(string=w946, offset (0)=9 ("偏移量(0)")) -> (substring=w940:string)  [unwired: 1 in]
        n473 = call "2转10进制字符串.vi"("二进制字符串"=w940) -> ("十进制数值"=w945:i32)
        n474 = Scale By Power Of 2(n=i16 23, x=sgl 1.0 ("长度（剩余）")) -> (x*2^n=w941:sgl)
        n475 = Divide(x=w945, y=w941) -> (x/y=w942:sgl)
        n476 = Add(x=w942, y=1.0) -> (x+y=w943:dbl)
        n477 = Multiply(x=w943, y=w939) -> (x*y=→"总累计流量":dbl)
      }
    }
    n478 = flat-sequence {
      frame #0 {
        n479 = case shown="真" "调零" {
          frame False {
          }
          frame True {
            n480 = local read "总累计流量"() -> (→"累计流量 2":dbl)
          }
        }
      }
      frame #1 {
        n481 = local read "总累计流量"() -> (w911:dbl)
        n482 = local read "累计流量 2"() -> (w910:dbl)
        n483 = Subtract(x=w911, y=w910) -> (x-y=→"调零后累计流量":dbl)
      }
    }
    n484 = local read "连接的字符串 4"() -> (w863:string)
    n485 = String To Byte Array(string=w863) -> (unsigned byte array=w865:u8[])
    n486 = Unbundle By Name("串口设置") -> ("波特率"=w891:u32, "数据位"=w890:u16, "校验"=w889:enum16{"None", "Odd", "Even", "Mark", "Space"}, "停止位"=w888:u16, "流控制"=w887:u16)
    n487 = for {
      shift-right: [w982] -> w864
      shift-left: "" -> [w984]
      tunnel: w865 -> [w991] mode=indexing
      n488 = Number To Hexadecimal String(2:w991) -> (0:w985:string)  [unwired: 1 in]
      n489 = String Length(string=w985) -> (length=w990:i32)
      n490 = Concatenate Strings("" ("字符串"), w985) -> (w986:string)
      n491 = Equal?(x=w990, y=2) -> (x = y?=w988:bool)
      n492 = Select(t=w985, s=w988, f=w986) -> (s? t:f=w983:string)
      n493 = Concatenate Strings(w984, w983) -> (w982:string)
    }
    "字符串 3" <- w864
    n494 = call-poly "VISA Configure Serial Port"("VISA resource name"="VISA资源名称", "baud rate (9600)"=w891, "data bits (8)"=w890, "parity (0:none)"=w889, "stop bits (10: 1 bit)"=w888, "flow control (0:none)"=w887) -> ("VISA resource name out"=w904:refnum<visa-resource-name>, "error out"=w905:errorcluster)  [unwired: 3 in, 5 out]
    n495 = VISA Write(VISA resource name=w904, write buffer="\u0005\u0003\u0000\u0000\u0000\u001a艆" ("Command"), error in (no error)=w905) -> (VISA resource name out=w898:refnum<visa-resource-name>, error out=w900:errorcluster)  [unwired: 1 out]
    n496 = flat-sequence {
      tunnel: w900 -> [w1003]
      tunnel: [w1003] -> w899
      tunnel: w898 -> [w1002]
      tunnel: [w1002] -> w897
      tunnel: "读取前延时(ms)" -> [w1004]
      frame #0 {
        n497 = Wait (ms)(milliseconds to wait=w1004) -> ()  [unwired: 1 out]
      }
    }
    n498 = property class="Instr"(reference=w897, error in=w899) -> (reference out=w895:refnum<visa-resource-name>, error out=w894:errorcluster, "Serial Settings:Number of Bytes at Serial Port"=w893:u32)
    "读取的字节" <- w893
    n499 = VISA Read(VISA resource name=w895, byte count=w893, error in (no error)=w894) -> (VISA resource name out=w902:refnum<visa-resource-name>, read buffer=w872:string, error out=w903:errorcluster)  [unwired: 1 out]
    "响应" <- w872
    n500 = String Subset(string=w872, offset (0)=51 ("偏移量(0)"), length (rest)=2 ("长度（剩余）")) -> (substring=w874:string)
    n501 = String Subset(string=w872, offset (0)=53 ("偏移量(0)"), length (rest)=2 ("长度（剩余）")) -> (substring=w875:string)
    n502 = String Subset(string=w872, offset (0)=5 ("偏移量(0)"), length (rest)=2 ("长度（剩余）")) -> (substring=w877:string)
    n503 = String Subset(string=w872, offset (0)=3 ("偏移量(0)"), length (rest)=2 ("长度（剩余）")) -> (substring=w876:string)
    n504 = Concatenate Strings(w875, w874) -> (→"连接的字符串 4":string)
    n505 = Concatenate Strings(w877, w876) -> (→"连接的字符串 3":string)
    n506 = VISA Close(VISA resource name=w902, error in (no error)=w903) -> (error out=w901:errorcluster)
    n507 = call <vilib>:"Simple Error Handler.vi"("error in (no error)"=w901) -> ()  [unwired: 1 in, 8 out]
  }
  n508 = stacked-sequence {
    frame #0 {
      w1007 = T4."Disabled and Grayed Out" ("禁用")
      w1008 = FALSE ("手动模式")
      w1005 = FALSE ("手动模式")
      w1006 = T4."Enabled" ("禁用")
      n509 = property on="调零" class="Bool"("DisabledEnum"=w1006) -> ()  [unwired: 2 in, 2 out]
      n510 = property on="紧急停止 2" class="Bool (严格)"("DisabledEnum"=w1006, "Value"=w1005) -> ()  [unwired: 2 in, 2 out]
      n511 = property on="手动模式" class="Bool (严格)"("DisabledEnum"=w1006, "Value"=w1005) -> ()  [unwired: 2 in, 2 out]
      n512 = property on="自动模式" class="Bool (严格)"("DisabledEnum"=w1006, "Value"=w1005) -> ()  [unwired: 2 in, 2 out]
      n513 = property on="紧急停止" class="Bool (严格)"("DisabledEnum"=w1006, "Value"=w1005) -> ()  [unwired: 2 in, 2 out]
      n514 = property on="数据保存 2" class="Bool (严格)"("Value"=w1005, "DisabledEnum"=w1006) -> ()  [unwired: 2 in, 2 out]
      n515 = property on="球阀预调确认" class="Bool (严格)"("DisabledEnum"=w1007, "Value"=w1008) -> ()  [unwired: 2 in, 2 out]
      n516 = property on="电磁阀2" class="Bool (严格)"("DisabledEnum"=w1007, "Value"=w1008) -> ()  [unwired: 2 in, 2 out]
      n517 = property on="试验结束" class="Bool (严格)"("Value"=w1008, "DisabledEnum"=w1007) -> ()  [unwired: 2 in, 2 out]
      n518 = property on="全部放气" class="Bool (严格)"("DisabledEnum"=w1007, "Value"=w1008) -> ()  [unwired: 2 in, 2 out]
      n519 = property on="保压时间固定" class="Bool (严格)"("DisabledEnum"=w1007, "Value"=w1008) -> ()  [unwired: 2 in, 2 out]
      n520 = property on="电磁阀1" class="Bool (严格)"("DisabledEnum"=w1007, "Value"=w1008) -> ()  [unwired: 2 in, 2 out]
      n521 = property on="试验结束 2" class="Bool (严格)"("DisabledEnum"=w1007, "Value"=w1008) -> ()  [unwired: 2 in, 2 out]
      n522 = property on="容器放气" class="Bool (严格)"("DisabledEnum"=w1007, "Value"=w1008) -> ()  [unwired: 2 in, 2 out]
      n523 = property on="放气" class="Bool (严格)"("DisabledEnum"=w1007, "Value"=w1008) -> ()  [unwired: 2 in, 2 out]
      n524 = property on="放气延迟" class="Bool (严格)"("DisabledEnum"=w1007, "Value"=w1008) -> ()  [unwired: 2 in, 2 out]
      n525 = property on="不保压" class="Bool (严格)"("DisabledEnum"=w1007, "Value"=w1008) -> ()  [unwired: 2 in, 2 out]
      n526 = property on="结束保存 2" class="Bool (严格)"("DisabledEnum"=w1007, "Value"=w1008) -> ()  [unwired: 2 in, 2 out]
      n527 = property on="球阀开口预调" class="DigNum (严格)"("DisabledEnum"=w1007) -> ()  [unwired: 2 in, 2 out]
      n528 = property on="p" class="DigNum (严格)"("DisabledEnum"=w1007) -> ()  [unwired: 2 in, 2 out]
      n529 = property on="D" class="DigNum (严格)"("DisabledEnum"=w1007) -> ()  [unwired: 2 in, 2 out]
      n530 = property on="I" class="DigNum (严格)"("DisabledEnum"=w1007) -> ()  [unwired: 2 in, 2 out]
      n531 = property on="cns" class="DigNum (严格)"("DisabledEnum"=w1007) -> ()  [unwired: 2 in, 2 out]
      n532 = property on="实验所需压力Mpa" class="DigNum (严格)"("DisabledEnum"=w1007) -> ()  [unwired: 2 in, 2 out]
      n533 = property on="球阀开口度" class="DigNum (严格)"("DisabledEnum"=w1007) -> ()  [unwired: 2 in, 2 out]
      n534 = property on="时间s" class="DigNum (严格)"("DisabledEnum"=w1007) -> ()  [unwired: 2 in, 2 out]
    }
    frame #1 {
      n535 = while {
        stop <- FALSE stop-if-true
        n536 = event shown="[7] \"试验结束 2\": 值改变" {
          selector: _ -> [_ _ _ _ _ _ _ _ _ _ _ _ _ _ _]
          dyn-events: _ -> [_ _ _ _ _ _ _ _ _ _ _ _ _ _ _]
          timeout: _ -> [_ _ _ _ _ _ _ _ _ _ _ _ _ _ _]
          event Timeout {
            n537 = event-data() -> ()  [unwired: 1 in, 3 out]
          }
          event "不保压": Value Change {
            n538 = event-data() -> ("NewVal"=w1016:bool)  [unwired: 1 in, 5 out]
            n539 = case shown="真" w1016 {
              tunnel: [T4."Enabled" ("禁用") w1023] -> w1015
              tunnel: [FALSE ("试验结束") _] -> w1013
              tunnel: [w1018 w1023] -> w1014
              tunnel: [w1018 T4."Enabled" ("禁用")] -> w1012
              tunnel: [w1018 T4."Enabled" ("禁用")] -> w1011
              tunnel: [FALSE ("球阀预调确认") _] -> w1010
              frame False {
                w1018 = T4."Disabled and Grayed Out" ("禁用")
              }
              frame True {
                w1023 = T4."Disabled and Grayed Out" ("禁用")
              }
            }
            n540 = property on="球阀开口预调" class="DigNum (严格)"("DisabledEnum"=w1011) -> ()  [unwired: 2 in, 2 out]
            n541 = property on="实验所需压力Mpa" class="DigNum (严格)"("DisabledEnum"=w1011) -> ()  [unwired: 2 in, 2 out]
            n542 = property on="球阀预调确认" class="Bool (严格)"("DisabledEnum"=w1011, "Value"=w1010) -> ()  [unwired: 2 in, 2 out]
            n543 = property on="试验结束 2" class="Bool (严格)"("Value"=w1013, "DisabledEnum"=w1012) -> ()  [unwired: 2 in, 2 out]
            n544 = property on="试验结束" class="Bool (严格)"("Value"=w1013, "DisabledEnum"=w1012) -> ()  [unwired: 2 in, 2 out]
            n545 = property on="保压时间固定" class="Bool (严格)"("DisabledEnum"=w1015) -> ()  [unwired: 2 in, 2 out]
            n546 = property on="放气延迟" class="Bool (严格)"("DisabledEnum"=w1015) -> ()  [unwired: 2 in, 2 out]
            n547 = property on="p" class="DigNum (严格)"("DisabledEnum"=w1014) -> ()  [unwired: 2 in, 2 out]
            n548 = property on="D" class="DigNum (严格)"("DisabledEnum"=w1014) -> ()  [unwired: 2 in, 2 out]
            n549 = property on="I" class="DigNum (严格)"("DisabledEnum"=w1014) -> ()  [unwired: 2 in, 2 out]
            n550 = property on="cns" class="DigNum (严格)"("DisabledEnum"=w1014) -> ()  [unwired: 2 in, 2 out]
            n551 = property on="时间s" class="DigNum (严格)"("DisabledEnum"=w1014) -> ()  [unwired: 2 in, 2 out]
          }
          event "放气延迟": Value Change {
            n552 = event-data() -> ("NewVal"=w1031:bool)  [unwired: 1 in, 5 out]
            n553 = case shown="假" w1031 {
              tunnel: [T4."Enabled" ("禁用") w1038] -> w1025
              tunnel: [FALSE ("试验结束") _] -> w1029
              tunnel: [w1032 w1038] -> w1030
              tunnel: [w1032 w1036] -> w1028
              tunnel: [w1032 T4."Enabled" ("禁用")] -> w1027
              tunnel: [FALSE ("球阀预调确认") _] -> w1026
              tunnel: [w1032 w1036] -> w1024
              frame False {
                w1032 = T4."Disabled and Grayed Out" ("禁用")
              }
              frame True {
                w1036 = T4."Enabled" ("禁用")
                w1038 = T4."Disabled and Grayed Out" ("禁用")
              }
            }
            n554 = property on="球阀开口预调" class="DigNum (严格)"("DisabledEnum"=w1027) -> ()  [unwired: 2 in, 2 out]
            n555 = property on="实验所需压力Mpa" class="DigNum (严格)"("DisabledEnum"=w1027) -> ()  [unwired: 2 in, 2 out]
            n556 = property on="球阀预调确认" class="Bool (严格)"("DisabledEnum"=w1027, "Value"=w1026) -> ()  [unwired: 2 in, 2 out]
            n557 = property on="试验结束 2" class="Bool (严格)"("Value"=w1029, "DisabledEnum"=w1028) -> ()  [unwired: 2 in, 2 out]
            n558 = property on="试验结束" class="Bool (严格)"("Value"=w1029, "DisabledEnum"=w1028) -> ()  [unwired: 2 in, 2 out]
            n559 = property on="保压时间固定" class="Bool (严格)"("DisabledEnum"=w1025) -> ()  [unwired: 2 in, 2 out]
            n560 = property on="p" class="DigNum (严格)"("DisabledEnum"=w1030) -> ()  [unwired: 2 in, 2 out]
            n561 = property on="D" class="DigNum (严格)"("DisabledEnum"=w1030) -> ()  [unwired: 2 in, 2 out]
            n562 = property on="I" class="DigNum (严格)"("DisabledEnum"=w1030) -> ()  [unwired: 2 in, 2 out]
            n563 = property on="cns" class="DigNum (严格)"("DisabledEnum"=w1030) -> ()  [unwired: 2 in, 2 out]
            n564 = property on="时间s" class="DigNum (严格)"("DisabledEnum"=w1024) -> ()  [unwired: 2 in, 2 out]
            n565 = property on="不保压" class="Bool (严格)"("DisabledEnum"=w1025) -> ()  [unwired: 2 in, 2 out]
          }
          event "保压时间固定": Value Change {
            n566 = event-data() -> ("NewVal"=w1043:bool)  [unwired: 1 in, 5 out]
            n567 = case shown="真" w1043 {
              tunnel: [w1046 w1048] -> w1042
              tunnel: [w1046 w1048] -> w1041
              tunnel: [T4."Disabled and Grayed Out" ("禁用") T4."Enabled" ("禁用")] -> w1039
              tunnel: [FALSE ("试验结束") _] -> w1040
              frame False {
                w1046 = T4."Enabled" ("禁用")
              }
              frame True {
                w1048 = T4."Disabled and Grayed Out" ("禁用")
              }
            }
            n568 = property on="试验结束 2" class="Bool (严格)"("Value"=w1040, "DisabledEnum"=w1039) -> ()  [unwired: 2 in, 2 out]
            n569 = property on="试验结束" class="Bool (严格)"("Value"=w1040, "DisabledEnum"=w1039) -> ()  [unwired: 2 in, 2 out]
            n570 = property on="实验所需压力Mpa" class="DigNum (严格)"("DisabledEnum"=w1039) -> ()  [unwired: 2 in, 2 out]
            n571 = property on="不保压" class="Bool (严格)"("DisabledEnum"=w1041) -> ()  [unwired: 2 in, 2 out]
            n572 = property on="放气延迟" class="Bool (严格)"("DisabledEnum"=w1042) -> ()  [unwired: 2 in, 2 out]
            n573 = property on="p" class="DigNum (严格)"("DisabledEnum"=w1039) -> ()  [unwired: 2 in, 2 out]
            n574 = property on="D" class="DigNum (严格)"("DisabledEnum"=w1039) -> ()  [unwired: 2 in, 2 out]
            n575 = property on="I" class="DigNum (严格)"("DisabledEnum"=w1039) -> ()  [unwired: 2 in, 2 out]
            n576 = property on="cns" class="DigNum (严格)"("DisabledEnum"=w1039) -> ()  [unwired: 2 in, 2 out]
            n577 = property on="时间s" class="DigNum (严格)"("DisabledEnum"=w1039) -> ()  [unwired: 2 in, 2 out]
          }
          event "手动模式": Value Change {
            n578 = event-data() -> ("NewVal"=w1053:bool)  [unwired: 1 in, 5 out]
            n579 = case shown="真" w1053 {
              tunnel: [w1056 w1059] -> w1049
              tunnel: [w1056 T4."Enabled" ("禁用")] -> w1054
              tunnel: [FALSE ("电磁阀2") _] -> w1052
              tunnel: [0.0 ("电控球阀 开口度") _] -> w1051
              tunnel: [T4."Enabled" ("禁用") w1059] -> w1050
              frame False {
                (unwired) T4."Disabled and Grayed Out" ("禁用")
                w1056 = T4."Disabled and Grayed Out" ("禁用")
              }
              frame True {
                w1059 = T4."Disabled and Grayed Out" ("禁用")
              }
            }
            n580 = property on="球阀开口度" class="DigNum (严格)"("Value"=w1051) -> ()  [unwired: 2 in, 2 out]
            n581 = property on="球阀开口度" class="DigNum (严格)"("DisabledEnum"=w1054) -> ()  [unwired: 2 in, 2 out]
            n582 = property on="电磁阀2" class="Bool (严格)"("DisabledEnum"=w1054, "Value"=w1052) -> ()  [unwired: 2 in, 2 out]
            n583 = property on="电磁阀1" class="Bool (严格)"("DisabledEnum"=w1054, "Value"=w1052) -> ()  [unwired: 2 in, 2 out]
            n584 = property on="自动模式" class="Bool (严格)"("DisabledEnum"=w1050) -> ()  [unwired: 2 in, 2 out]
            n585 = property on="试验结束" class="Bool (严格)"("DisabledEnum"=w1049) -> ()  [unwired: 2 in, 2 out]
            n586 = property on="实验所需压力Mpa" class="DigNum (严格)"("DisabledEnum"=w1049) -> ()  [unwired: 2 in, 2 out]
            n587 = property on="cns" class="DigNum (严格)"("DisabledEnum"=w1049) -> ()  [unwired: 2 in, 2 out]
            n588 = property on="不保压" class="Bool (严格)"("DisabledEnum"=w1049) -> ()  [unwired: 2 in, 2 out]
            n589 = property on="放气" class="Bool (严格)"("DisabledEnum"=w1049) -> ()  [unwired: 2 in, 2 out]
            n590 = property on="保压时间固定" class="Bool (严格)"("DisabledEnum"=w1049) -> ()  [unwired: 2 in, 2 out]
            n591 = property on="放气延迟" class="Bool (严格)"("DisabledEnum"=w1049) -> ()  [unwired: 2 in, 2 out]
            n592 = property on="p" class="DigNum (严格)"("DisabledEnum"=w1049) -> ()  [unwired: 2 in, 2 out]
            n593 = property on="D" class="DigNum (严格)"("DisabledEnum"=w1049) -> ()  [unwired: 2 in, 2 out]
            n594 = property on="I" class="DigNum (严格)"("DisabledEnum"=w1049) -> ()  [unwired: 2 in, 2 out]
            n595 = property on="时间s" class="DigNum (严格)"("DisabledEnum"=w1049) -> ()  [unwired: 2 in, 2 out]
            n596 = property on="容器放气" class="Bool (严格)"("DisabledEnum"=w1049) -> ()  [unwired: 2 in, 2 out]
            n597 = property on="全部放气" class="Bool (严格)"("DisabledEnum"=w1049) -> ()  [unwired: 2 in, 2 out]
            n598 = property on="不保压" class="Bool (严格)"("DisabledEnum"=w1049) -> ()  [unwired: 2 in, 2 out]
            n599 = property on="试验结束 2" class="Bool (严格)"("DisabledEnum"=w1049) -> ()  [unwired: 2 in, 2 out]
          }
          event "自动模式": Value Change {
            n600 = event-data() -> ("NewVal"=w1070:bool)  [unwired: 1 in, 5 out]
            n601 = case shown="真" w1070 {
              tunnel: [w1072 T4."Enabled" ("禁用")] -> w1064
              tunnel: [w1072 w1074] -> w1065
              tunnel: [w1071 _] -> w1063
              tunnel: [_ FALSE ("电磁阀2")] -> w1069
              tunnel: [w1072 w1074] -> w1062
              tunnel: [w1072 w1074] -> w1068
              tunnel: [T4."Enabled" ("禁用") w1074] -> w1067
              tunnel: [w1071 _] -> w1066
              tunnel: [w1071 _] -> w1061
              frame False {
                w1071 = FALSE ("保压时间非固定")
                w1072 = T4."Disabled and Grayed Out" ("禁用")
              }
              frame True {
                w1074 = T4."Disabled and Grayed Out" ("禁用")
              }
            }
            n602 = property on="试验结束" class="Bool (严格)"("Value"=w1066, "DisabledEnum"=w1065) -> ()  [unwired: 2 in, 2 out]
            n603 = property on="试验结束 2" class="Bool (严格)"("Value"=w1066, "DisabledEnum"=w1065) -> ()  [unwired: 2 in, 2 out]
            n604 = property on="球阀开口度" class="DigNum (严格)"("DisabledEnum"=w1065) -> ()  [unwired: 2 in, 2 out]
            n605 = property on="实验所需压力Mpa" class="DigNum (严格)"("DisabledEnum"=w1068) -> ()  [unwired: 2 in, 2 out]
            n606 = property on="cns" class="DigNum (严格)"("DisabledEnum"=w1068) -> ()  [unwired: 2 in, 2 out]
            n607 = property on="电磁阀2" class="Bool (严格)"("DisabledEnum"=w1065, "Value"=w1069) -> ()  [unwired: 2 in, 2 out]
            n608 = property on="电磁阀1" class="Bool (严格)"("DisabledEnum"=w1065, "Value"=w1069) -> ()  [unwired: 2 in, 2 out]
            n609 = property on="手动模式" class="Bool (严格)"("DisabledEnum"=w1067) -> ()  [unwired: 2 in, 2 out]
            n610 = property on="放气延迟" class="Bool (严格)"("DisabledEnum"=w1064, "Value"=w1063) -> ()  [unwired: 2 in, 2 out]
            n611 = property on="保压时间固定" class="Bool (严格)"("DisabledEnum"=w1064, "Value"=w1063) -> ()  [unwired: 2 in, 2 out]
            n612 = property on="不保压" class="Bool (严格)"("DisabledEnum"=w1064, "Value"=w1063) -> ()  [unwired: 2 in, 2 out]
            n613 = property on="球阀开口预调" class="DigNum (严格)"("DisabledEnum"=w1062) -> ()  [unwired: 2 in, 2 out]
            n614 = property on="全部放气" class="Bool (严格)"("DisabledEnum"=w1062, "Value"=w1063) -> ()  [unwired: 2 in, 2 out]
            n615 = property on="容器放气" class="Bool (严格)"("DisabledEnum"=w1062, "Value"=w1063) -> ()  [unwired: 2 in, 2 out]
            n616 = property on="p" class="DigNum (严格)"("DisabledEnum"=w1062) -> ()  [unwired: 2 in, 2 out]
            n617 = property on="D" class="DigNum (严格)"("DisabledEnum"=w1062) -> ()  [unwired: 2 in, 2 out]
            n618 = property on="I" class="DigNum (严格)"("DisabledEnum"=w1062) -> ()  [unwired: 2 in, 2 out]
            n619 = property on="时间s" class="DigNum (严格)"("DisabledEnum"=w1062) -> ()  [unwired: 2 in, 2 out]
            n620 = property on="球阀预调确认" class="Bool (严格)"("Value"=w1061, "DisabledEnum"=w1062) -> ()  [unwired: 2 in, 2 out]
            n621 = property on="放气" class="Bool (严格)"("DisabledEnum"=w1064, "Value"=w1063) -> ()  [unwired: 2 in, 2 out]
          }
          event "试验结束": Value Change {
            n622 = event-data() -> ("NewVal"=w1078:bool)  [unwired: 1 in, 5 out]
            n623 = property on="试验结束 2" class="Bool (严格)"("Value"=w1078) -> ()  [unwired: 2 in, 2 out]
            n624 = case shown="假" w1078 {
              tunnel: [T4."Enabled" ("禁用") T4."Disabled and Grayed Out" ("禁用")] -> w1079
              tunnel: [_ FALSE ("放气")] -> w1077
              frame False {
              }
              frame True {
              }
            }
            n625 = property on="全部放气" class="Bool (严格)"("DisabledEnum"=w1079, "Value"=w1077) -> ()  [unwired: 2 in, 2 out]
            n626 = property on="放气" class="Bool (严格)"("DisabledEnum"=w1079, "Value"=w1077) -> ()  [unwired: 2 in, 2 out]
            n627 = property on="容器放气" class="Bool (严格)"("DisabledEnum"=w1079, "Value"=w1077) -> ()  [unwired: 2 in, 2 out]
          }
          event "试验结束 2": Value Change {
            n628 = event-data() -> ("NewVal"=w1083:bool)  [unwired: 1 in, 5 out]
            n629 = property on="试验结束" class="Bool (严格)"("Value"=w1083) -> ()  [unwired: 2 in, 2 out]
            n630 = case shown="真" w1083 {
              tunnel: [T4."Enabled" ("禁用") T4."Disabled and Grayed Out" ("禁用")] -> w1085
              tunnel: [_ FALSE ("放气")] -> w1084
              frame False {
              }
              frame True {
              }
            }
            n631 = property on="全部放气" class="Bool (严格)"("DisabledEnum"=w1085, "Value"=w1084) -> ()  [unwired: 2 in, 2 out]
            n632 = property on="放气" class="Bool (严格)"("DisabledEnum"=w1085, "Value"=w1084) -> ()  [unwired: 2 in, 2 out]
            n633 = property on="容器放气" class="Bool (严格)"("DisabledEnum"=w1085, "Value"=w1084) -> ()  [unwired: 2 in, 2 out]
          }
          event "放气": Value Change {
            n634 = event-data() -> ("NewVal"=w1091:bool)  [unwired: 1 in, 5 out]
            n635 = case shown="假" w1091 {
              tunnel: [T4."Disabled and Grayed Out" ("禁用") T4."Enabled" ("禁用")] -> w1090
              tunnel: [FALSE ("容器放气") _] -> w1089
              frame False {
              }
              frame True {
              }
            }
            n636 = property on="容器放气" class="Bool (严格)"("DisabledEnum"=w1090, "Value"=w1089) -> ()  [unwired: 2 in, 2 out]
            n637 = property on="全部放气" class="Bool (严格)"("DisabledEnum"=w1090, "Value"=w1089) -> ()  [unwired: 2 in, 2 out]
          }
          event "全部放气": Value Change {
            n638 = event-data() -> ("NewVal"=w1096:bool)  [unwired: 1 in, 5 out]
            n639 = case shown="假" w1096 {
              tunnel: [T4."Enabled" ("禁用") T4."Disabled and Grayed Out" ("禁用")] -> w1095
              frame False {
              }
              frame True {
              }
            }
            n640 = property on="容器放气" class="Bool (严格)"("DisabledEnum"=w1095) -> ()  [unwired: 2 in, 2 out]
          }
          event "容器放气": Value Change {
            n641 = event-data() -> ("NewVal"=w1100:bool)  [unwired: 1 in, 5 out]
            n642 = case shown="假" w1100 {
              tunnel: [T4."Enabled" ("禁用") T4."Disabled and Grayed Out" ("禁用")] -> w1099
              frame False {
              }
              frame True {
              }
            }
            n643 = property on="全部放气" class="Bool (严格)"("DisabledEnum"=w1099) -> ()  [unwired: 2 in, 2 out]
          }
          event "紧急停止": Value Change {
            n644 = event-data() -> ("NewVal"=w1103:bool)  [unwired: 1 in, 5 out]
            n645 = property on="紧急停止 2" class="Bool (严格)"("Value"=w1103) -> ()  [unwired: 2 in, 2 out]
          }
          event "紧急停止 2": Value Change {
            n646 = event-data() -> ("NewVal"=w1104:bool)  [unwired: 1 in, 5 out]
            n647 = property on="紧急停止" class="Bool (严格)"("Value"=w1104) -> ()  [unwired: 2 in, 2 out]
          }
          event "数据保存 2": Value Change {
            n648 = event-data() -> ("NewVal"=w1106:bool)  [unwired: 1 in, 5 out]
            n649 = case shown="假" w1106 {
              tunnel: [T4."Disabled and Grayed Out" ("禁用") T4."Enabled" ("禁用")] -> w1105
              frame False {
              }
              frame True {
              }
            }
            n650 = property on="结束保存 2" class="Bool (严格)"("DisabledEnum"=w1105) -> ()  [unwired: 2 in, 2 out]
          }
          event "结束保存 2": Value Change {
            n651 = event-data() -> ("NewVal"=w1111:bool)  [unwired: 1 in, 5 out]
            n652 = case shown="真" w1111 {
              tunnel: [_ FALSE ("数据保存 2")] -> w1110
              tunnel: [T4."Enabled" ("禁用") T4."Disabled and Grayed Out" ("禁用")] -> w1109
              frame False {
              }
              frame True {
              }
            }
            n653 = property on="数据保存 2" class="Bool (严格)"("Value"=w1110, "DisabledEnum"=w1109) -> ()  [unwired: 2 in, 2 out]
          }
        }
      }
    }
  }
